vi "tvac_gui_chamber.vi"() -> ()   [LabVIEW 2016]
uses:
  <vilib>/httpClient/LabVIEWHTTPClient.lvlib
  <vilib>/httpClient/ClientHandle.ctl
  msg7171_linux.llb/send single message.vi
  <vilib>/httpClient/POSTBuffer.vi
panel:
  out "headers":string
  in  "ThermalProfile":bool
  in  "Read Zones":bool
  out "value":cluster{"ZoneSetPoint":dbl[], "ZoneTemp":dbl[]}
  out "output cluster":T1
  out "Cluster":T2
  in  "Custom Graph Selector":i32
  in  "exit":bool
  in  "AlarmColor":u32(colorbox)
  in  "Alarm String":string
  in  "Plot Color":u32(colorbox)=16860
  in  "Temperature":dbl format="%#_13g"
  in  "TC Label":string
  in  "Graph ON/OFF":u32(colorbox)=4250624
  in  "index (col)":i32
  in  "index (row)":i32
  out "working array":bool[](array[boolean])
  in  "Local Debug":bool
  in  "Tab Control":enum32{"TCs", "Graphs", "Thermal Profile"}(tab)
  in  "Log/Linear Y-Axis":u16(ring) items=["Linear", "Log"]
  in  "Total Time":dbl
  in  "Set Time TC Graph":bool
  in  "Graphing Selection":u16(ring) items=["User Selection", "Graph All Thermocouples", "Clear Graph"]
  in  "Time Scale":u16(ring) items=["Minutes", "Hours", "Seconds"]
  out "Waveform Chart":waveform(dbl)[](graph)
  out "Thermocouples":T3(array[cluster])
  in  "Log/Linear Y-Axis 6":u16(ring) items=["Linear", "Log"]
  in  "Log/Linear Y-Axis 5":u16(ring) items=["Linear", "Log"]
  in  "Log/Linear Y-Axis 3":u16(ring) items=["Linear", "Log"]
  in  "Log/Linear Y-Axis 2":u16(ring) items=["Linear", "Log"]
  in  "Total Time 6":dbl
  in  "Set Time TC Graph 6":bool
  in  "Time Scale 6":u16(ring) items=["Minutes", "Hours", "Seconds"]
  in  "Total Time 5":dbl
  in  "Set Time TC Graph 5":bool
  in  "Time Scale 5":u16(ring) items=["Minutes", "Hours", "Seconds"]
  in  "Total Time 4":dbl
  in  "Set Time TC Graph 4":bool
  in  "Time Scale 4":u16(ring) items=["Minutes", "Hours", "Seconds"]
  in  "Total Time 3":dbl
  in  "Set Time TC Graph 3":bool
  in  "Time Scale 3":u16(ring) items=["Minutes", "Hours", "Seconds"]
  in  "Total Time 2":dbl
  in  "Set Time TC Graph 2":bool
  in  "Time Scale 2":u16(ring) items=["Minutes", "Hours", "Seconds"]
  in  "Log/Linear Y-Axis 1":u16(ring) items=["Linear", "Log"]
  in  "Total Time 1":dbl
  in  "Set Time TC Graph 1":bool
  in  "Time Scale 1":u16(ring) items=["Minutes", "Hours", "Seconds"]
  in  "Custom Chart 2 Selection":i32[](listbox)=[0]
  in  "Custom Chart 1 Selection":i32[](listbox)=[0]
  out "Custom Chart 1":waveform(dbl)[](graph)
  in  "Custom Chart 3 Selection":i32[](listbox)=[0]
  in  "Custom Chart 4 Selection":i32[](listbox)=[0]
  in  "Custom Chart 5 Selection":i32[](listbox)=[0]
  in  "Custom Chart 6 Selection":i32[](listbox)=[0]
  out "Custom Chart 2":waveform(dbl)[](graph)
  out "Custom Chart 3":waveform(dbl)[](graph)
  out "Custom Chart 4":waveform(dbl)[](graph)
  out "Custom Chart 5":waveform(dbl)[](graph)
  out "Custom Chart 6":waveform(dbl)[](graph)
  in  "Log/Linear Y-Axis 4":u16(ring) items=["Linear", "Log"]
  in  "Run Profile 2":bool
  in  "Run Profile":bool
  in  "Resume Profile":bool
  in  "Stop Profile":bool
  in  "Pause Profile":bool
  in  "Hold Profile":bool
  in  "Set Z 1":bool
  in  "Z3 Thermal Profile":i32(listbox)
  in  "Z2 Thermal Profile":i32(listbox)
  in  "Z1 Thermal Profile":i32(listbox)
  in  "Zone 3 Temp":u16(ring) items=["Average", "Minimum", "Maximum"]
  in  "Zone 2 Temp":u16(ring) items=["Average", "Minimum", "Maximum"]
  in  "Zone 1 Temp":u16(ring) items=["Average", "Minimum", "Maximum"]
  in  "Zone 1 TC":i32[](listbox)=[0]
  in  "Zone 2 TC":i32[](listbox)=[0]
  in  "Zone 3 TC":i32[](listbox)=[0]
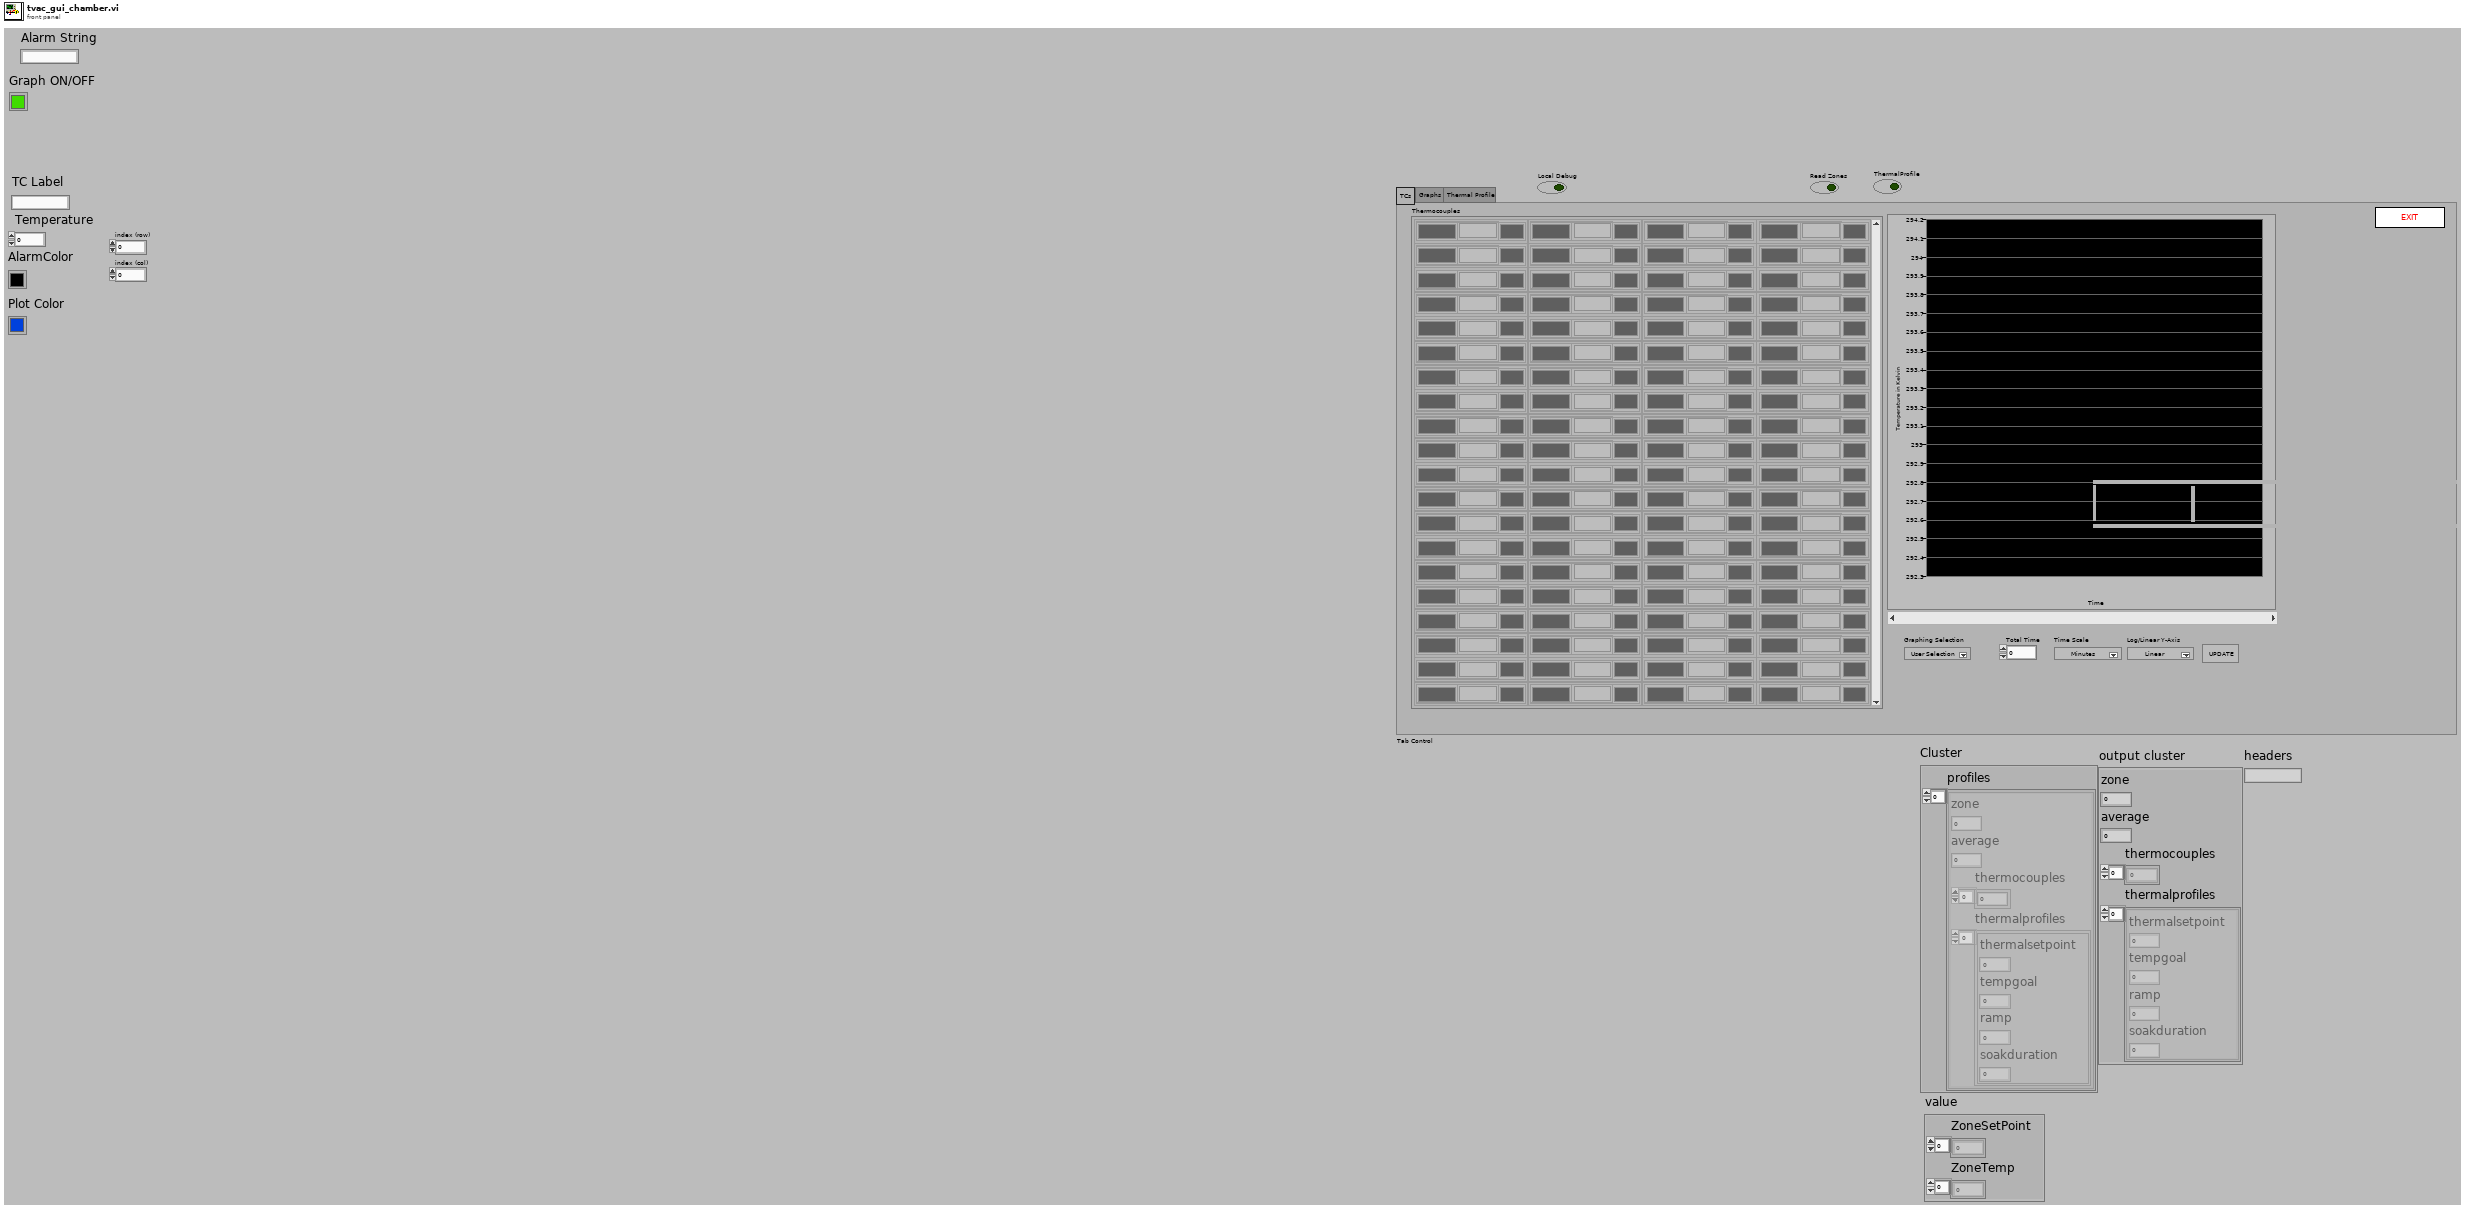
[diagram p1: front panel]
types:
  T1 = cluster{"zone":i32, "average":i32, "thermocouples":dbl[], "thermalprofiles":cluster{"thermalsetpoint":i32, "tempgoal":i32, "ramp":i32, "soakduration":i32}[]}
  T2 = cluster{"profiles":cluster{"zone":i32, "average":i32, "thermocouples":dbl[], "thermalprofiles":cluster{"thermalsetpoint":i32, "tempgoal":i32, "ramp":i32, "soakduration":i32}[]}[]}
  T3 = cluster{"TC Label":string, "Alarm Status":string, "Alarm Color":u32, "Temperature":string, "PlotColor":u32, "Graph On/Off":u32}[][]
  T4 = cluster{"thermocouple":i32, "time":dbl, "temp":dbl, "working":bool, "alarm":i32}[]
  T5 = cluster{"Cp Stage 1 Temp":dbl[], "Cp Stage 2 Temp":dbl[], "Compressor Temp":dbl[]}
  T6 = typedef "LabVIEWHTTPClient.lvlib/ClientHandle.ctl" = refnum<k1>
  T7 = cluster{"go":bool, "Http session":T6, "URL prefex":string, "index (row)":i32, "index (col)":i32, "Graph ON/OFF":u32, "TC Label":string, "Temperature":dbl, "AlarmColor":u32, "Plot Color":u32, "Alarm String":string, "Thermocouples":cluster{"TC Label":string, "Alarm Status":string, "Alarm Color":u32, "Temperature":string, "PlotColor":u32, "Graph On/Off":u32}[][], "working array":bool[], "i":i32, "NumberTCs":i32, "Waveform Chart":waveform(dbl)[], "Custom Chart 1":waveform(dbl)[], "Pressure":dbl[], "numSensors":i32, "Database":dbl[], "PumpTemps":cluster{"Cp Stage 1 Temp":dbl[], "Cp Stage 2 Temp":dbl[], "Compressor Temp":dbl[]}, "Zones":dbl[], "Time":i32, "TCs":cluster{"thermocouple":i32, "time":dbl, "temp":dbl, "working":bool, "alarm":i32}[]}
  T8 = cluster{"TC Label":string, "Alarm Status":string, "Alarm Color":u32, "Temperature":string, "PlotColor":u32, "Graph On/Off":u32}
  T9 = cluster{"CryoPressure":dbl, "ChamberPressure":dbl, "RoughingPressure":dbl}
  T10 = cluster{"time":string, "TCs":cluster{"thermocouple":i32, "time":dbl, "temp":dbl, "working":bool, "alarm":i32}[]}
  T11 = cluster{"DutyCycle":i32, "Stage1Temp":i32, "CryoPumpReadyState":cluster{"MotorOn":bool, "Ready":bool}, "PurgeValveState":bool, "RegenError":string, "RegenStep":string, "RoughingValveState":bool, "RoughingInterlock":cluster{"RoughingPermission":bool, "RoughingNeeded":bool, "Cryopumprunning":bool}, "Stage2Temp":i32, "Status":cluster{"PumpOn":bool, "RoughOpen":bool, "PurgeOpen":bool, "ThermocoupleGaugeOn":bool, "PowerFailureOccurred":bool}, "TcPressure":i32}
  T12 = typedef "LVPositionTypeDef.ctl" = cluster{"Left":i32, "Top":i32}
  T13 = typedef "LVPoint32TypeDef.ctl" = cluster{"Horizontal":i32, "Vertical":i32}
  T14 = typedef "LVRangeTypeDef.ctl" = cluster{"Minimum":dbl, "Maximum":dbl, "Increment":dbl, "Minor Increment":dbl, "Start":dbl}
  T15 = cluster{"zone":i32, "average":i32, "thermocouples":dbl[], "thermalprofiles":cluster{"thermalsetpoint":i32, "tempgoal":i32, "ramp":i32, "soakduration":i32}[]}[]
  T16 = cluster{"profiles[0]":cluster{"zone":i32, "average":i32, "thermocouples":dbl[], "thermalprofiles":cluster{"thermalsetpoint":i32, "tempgoal":i32, "ramp":i32, "soakduration":i32}[]}, "profiles[1]":cluster{"zone":i32, "average":i32, "thermocouples":dbl[], "thermalprofiles":cluster{"thermalsetpoint":i32, "tempgoal":i32, "ramp":i32, "soakduration":i32}[]}, "profiles[2]":cluster{"zone":i32, "average":i32, "thermocouples":dbl[], "thermalprofiles":cluster{"thermalsetpoint":i32, "tempgoal":i32, "ramp":i32, "soakduration":i32}[]}, "profiles[3]":cluster{"zone":i32, "average":i32, "thermocouples":dbl[], "thermalprofiles":cluster{"thermalsetpoint":i32, "tempgoal":i32, "ramp":i32, "soakduration":i32}[]}, "profiles[4]":cluster{"zone":i32, "average":i32, "thermocouples":dbl[], "thermalprofiles":cluster{"thermalsetpoint":i32, "tempgoal":i32, "ramp":i32, "soakduration":i32}[]}, "profiles[5]":cluster{"zone":i32, "average":i32, "thermocouples":dbl[], "thermalprofiles":cluster{"thermalsetpoint":i32, "tempgoal":i32, "ramp":i32, "soakduration":i32}[]}, "profiles[6]":cluster{"zone":i32, "average":i32, "thermocouples":dbl[], "thermalprofiles":cluster{"thermalsetpoint":i32, "tempgoal":i32, "ramp":i32, "soakduration":i32}[]}, "profiles[7]":cluster{"zone":i32, "average":i32, "thermocouples":dbl[], "thermalprofiles":cluster{"thermalsetpoint":i32, "tempgoal":i32, "ramp":i32, "soakduration":i32}[]}, "profiles[8]":cluster{"zone":i32, "average":i32, "thermocouples":dbl[], "thermalprofiles":cluster{"thermalsetpoint":i32, "tempgoal":i32, "ramp":i32, "soakduration":i32}[]}}
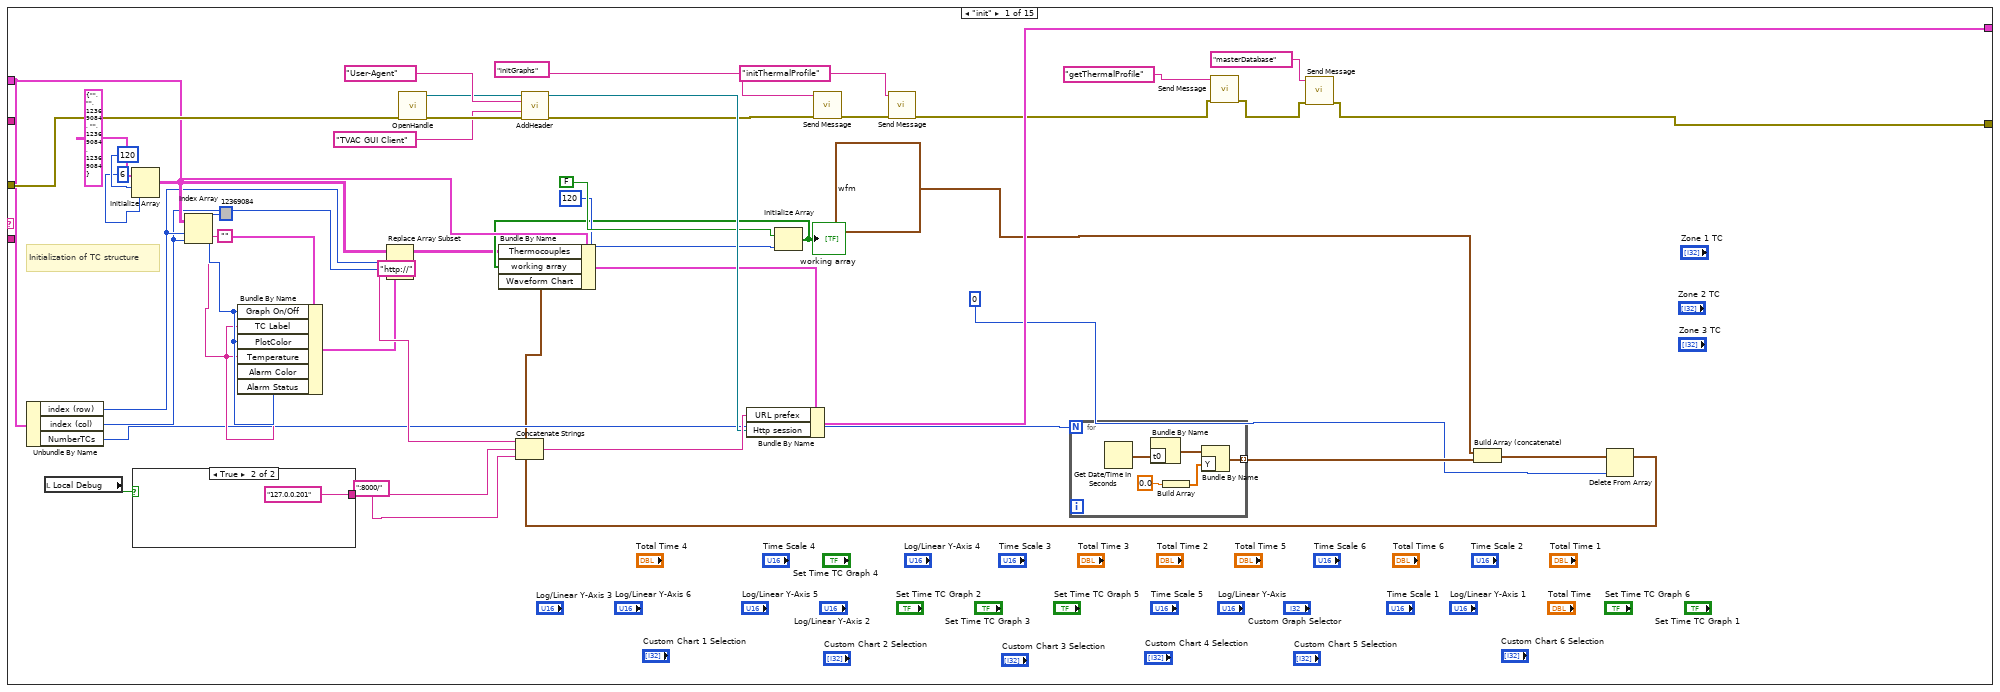
[diagram p2: hidden frame]
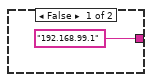
[diagram p3: hidden frame]
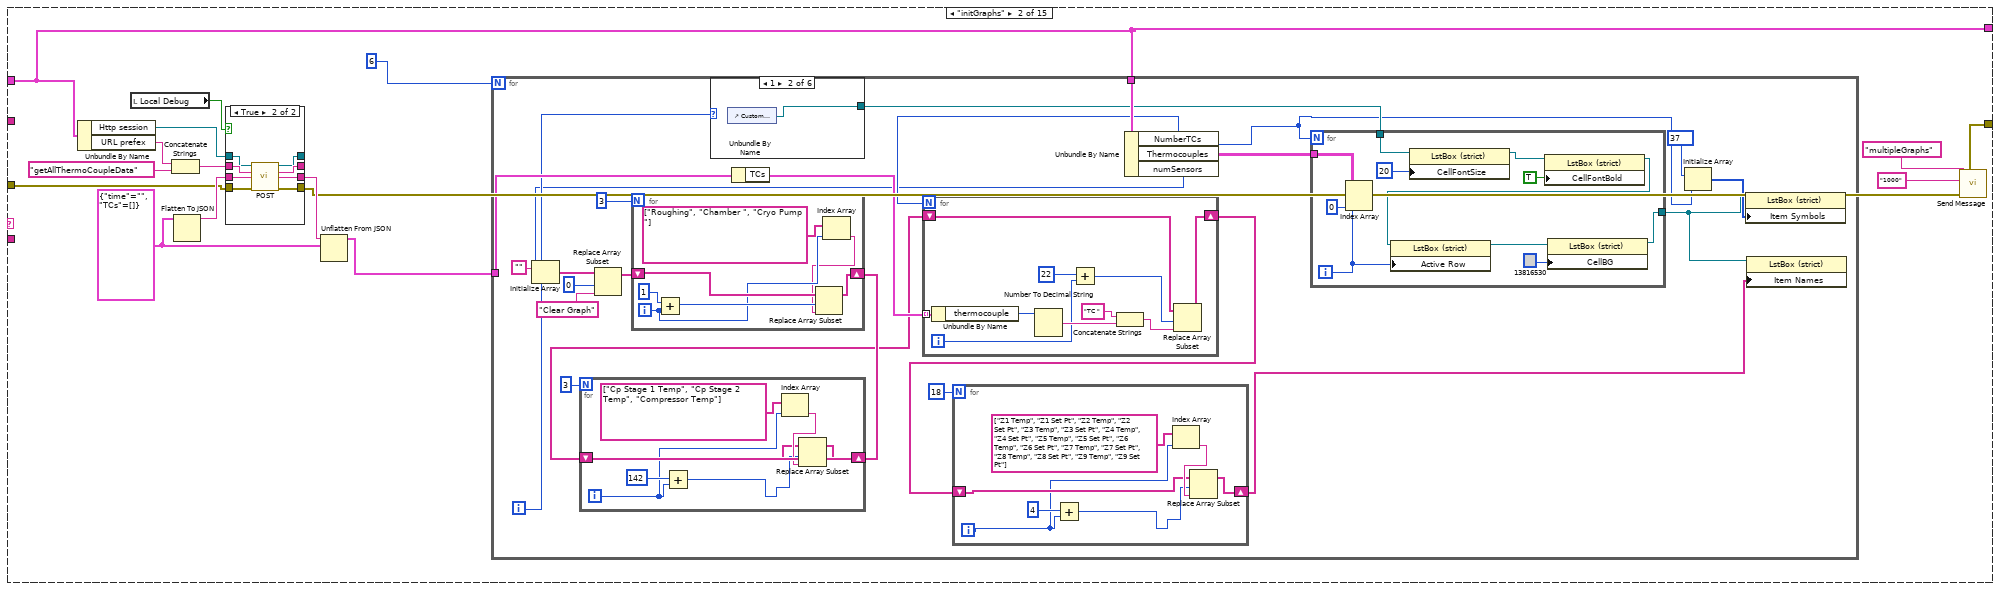
[diagram p4: hidden frame]
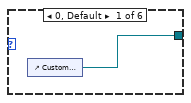
[diagram p5: hidden frame]
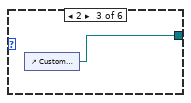
[diagram p6: hidden frame]
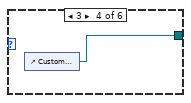
[diagram p7: hidden frame]
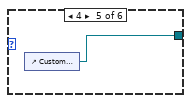
[diagram p8: hidden frame]
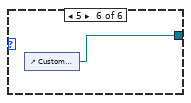
[diagram p9: hidden frame]
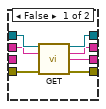
[diagram p10: hidden frame]
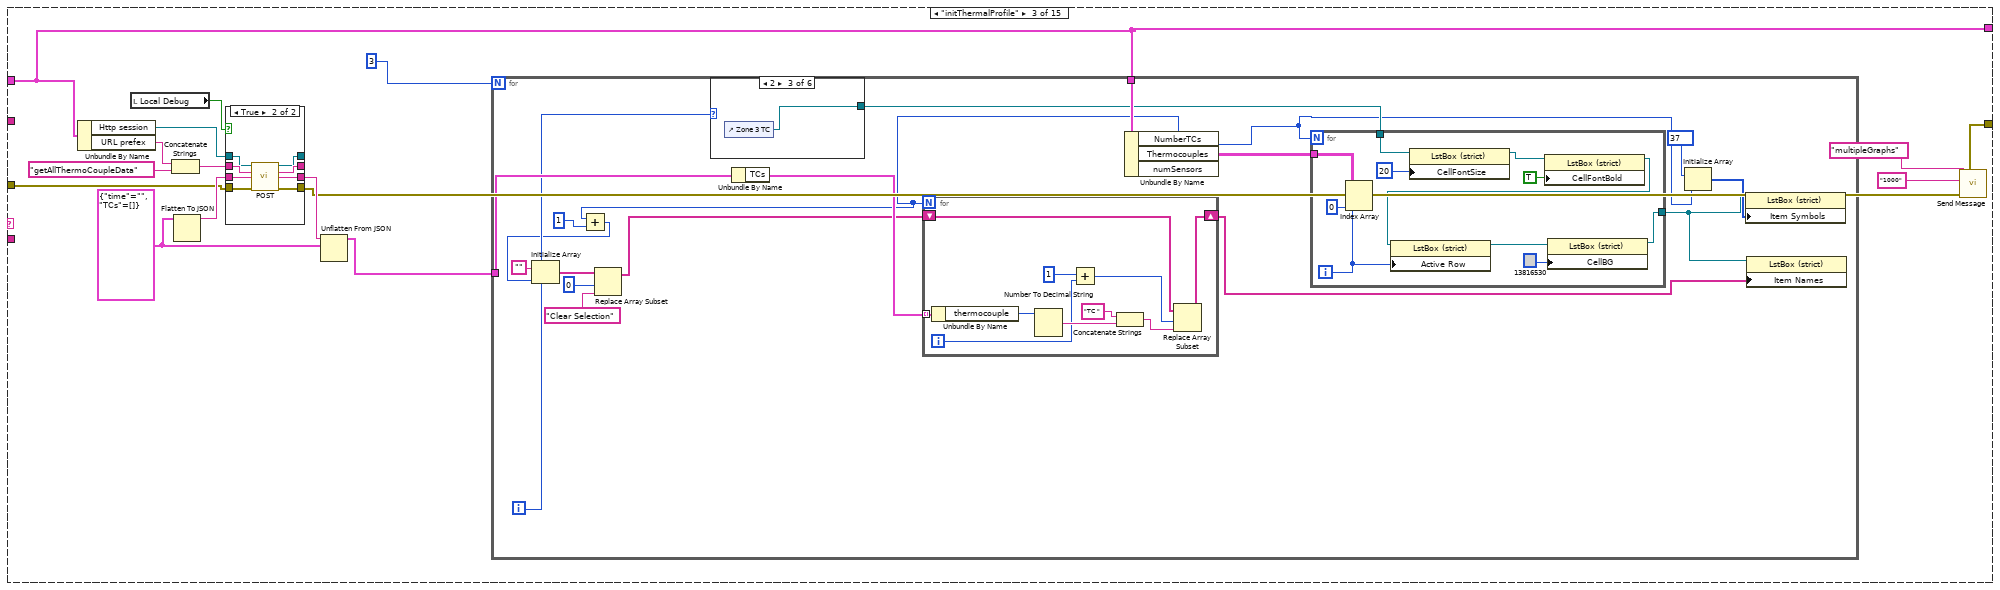
[diagram p11: hidden frame]
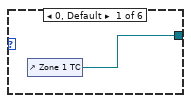
[diagram p12: hidden frame]
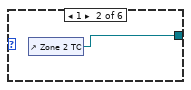
[diagram p13: hidden frame]
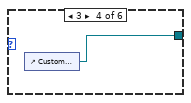
[diagram p14: hidden frame]
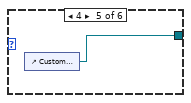
[diagram p15: hidden frame]
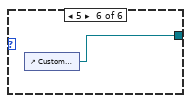
[diagram p16: hidden frame]
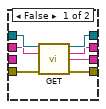
[diagram p17: hidden frame]
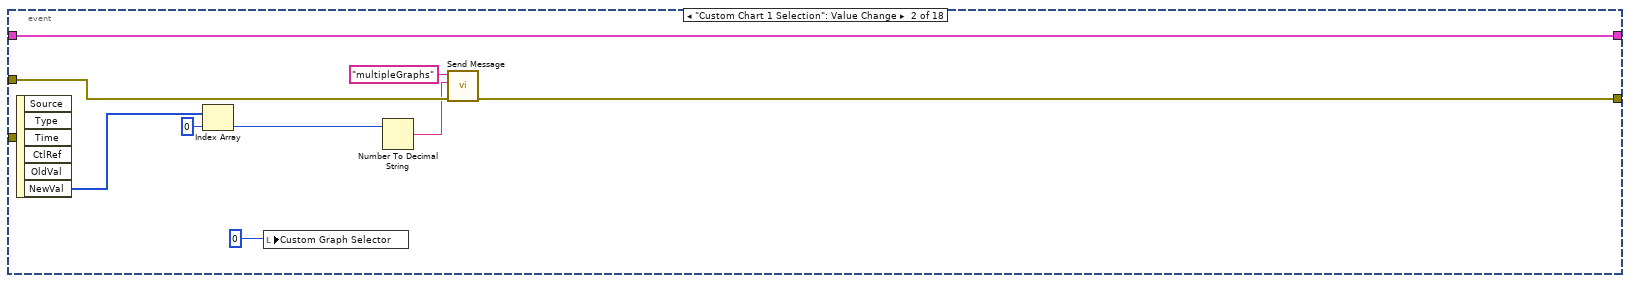
[diagram p18: hidden frame]
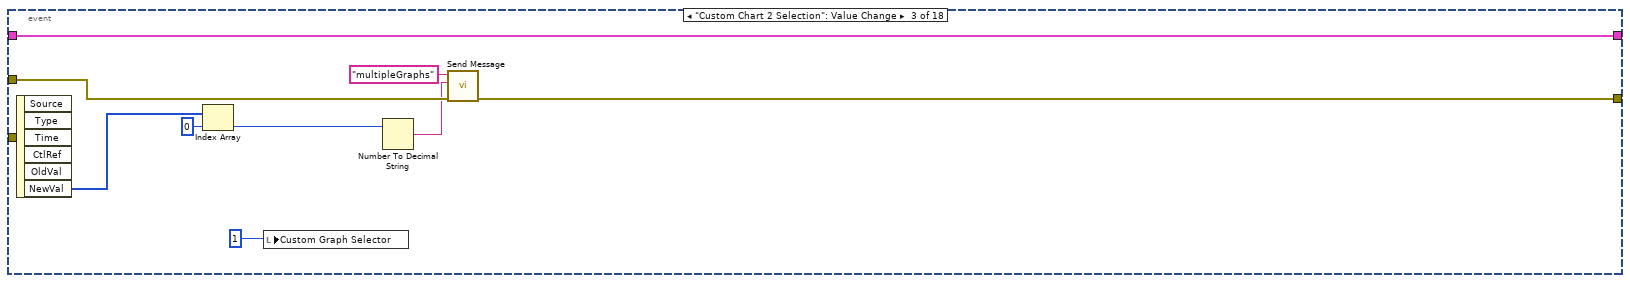
[diagram p19: hidden frame]
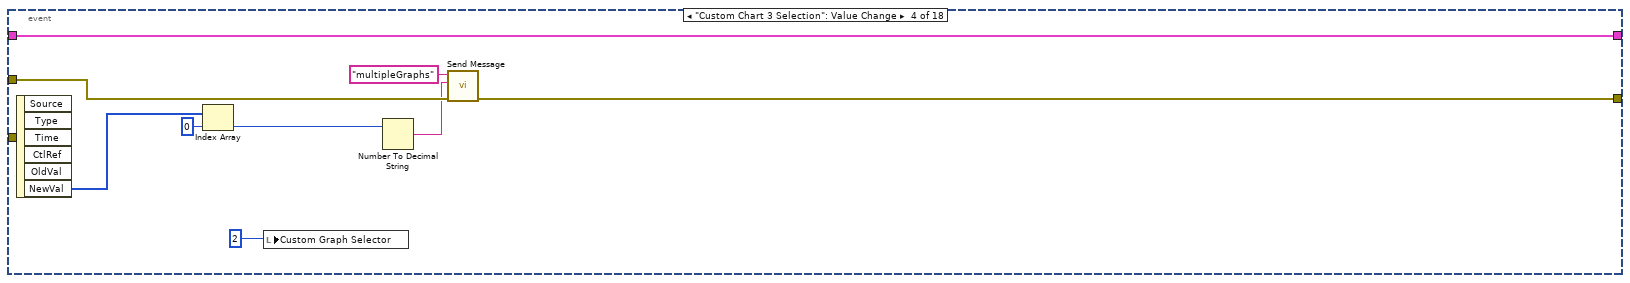
[diagram p20: hidden frame]
diagram:
  w5 = T5 {"Cp Stage 1 Temp"=[0.0], "Cp Stage 2 Temp"=[0.0], "Compressor Temp"=[0.0]}  # PumpTemps
  w8 = dbl[] [0.0, 0.0, 0.0]  # Pressure
  w28 = ""  # URL prefex
  w29 = T6 refnum  # Http session
  w30 = TRUE  # go
  n1 = call "Register Module.vi"() -> ("error out"=w26:errorcluster)  [unwired: 10 in, 1 out]
  n2 = call-poly "Send Message.vi"("error in (no error)"=w26, "event"="init") -> ("error out"=w25:errorcluster)  [unwired: 9 in]
  n3 = local read "Waveform Chart"() -> (w12:waveform(dbl)[])
  n4 = local read "Thermocouples"() -> (w10:T3)
  n5 = local read "Custom Chart 1"() -> (w9:waveform(dbl)[])
  n6 = Bundle("go"=w30, "Http session"=w29, "URL prefex"=w28, "index (row)"="index (row)", "index (col)"="index (col)", "Graph ON/OFF"="Graph ON/OFF", "TC Label"="TC Label", "Temperature"="Temperature", "AlarmColor"="AlarmColor", "Plot Color"="Plot Color", "Alarm String"="Alarm String", "Thermocouples"=w10, "working array"=bool[] [TRUE, TRUE, TRUE, TRUE, TRUE, TRUE, TRUE, TRUE, TRUE, TRUE, TRUE, TRUE, TRUE, TRUE, TRUE, TRUE, TRUE, TRUE, TRUE, TRUE, TRUE, TRUE, TRUE, TRUE, TRUE, TRUE, TRUE, TRUE, TRUE, TRUE, TRUE, TRUE, TRUE, TRUE, TRUE, TRUE, TRUE, TRUE, TRUE, TRUE, TRUE, TRUE, TRUE, TRUE, TRUE, TRUE, TRUE, TRUE, TRUE, TRUE, TRUE, TRUE, TRUE, TRUE, TRUE, TRUE, TRUE, TRUE, TRUE, TRUE, TRUE, TRUE, TRUE, TRUE, TRUE, TRUE, TRUE, TRUE, TRUE, TRUE, TRUE, TRUE, TRUE, TRUE, TRUE, TRUE, TRUE, TRUE, TRUE, TRUE, TRUE, TRUE, TRUE, TRUE, TRUE, TRUE, TRUE, TRUE, TRUE, TRUE, TRUE, TRUE, TRUE, TRUE, TRUE, TRUE, TRUE, TRUE, TRUE, TRUE, TRUE, TRUE, TRUE, TRUE, TRUE, TRUE, TRUE, TRUE, TRUE, TRUE, TRUE, TRUE, TRUE, TRUE, TRUE, TRUE, TRUE, TRUE, TRUE, TRUE], "i"=0, "NumberTCs"=120, "Waveform Chart"=w12, "Custom Chart 1"=w9, "Pressure"=w8, "numSensors"=145, "Database"=dbl[] [0.0, 1000.5841582194602, 1000.5841582194602, 1000.5841582194602, 0.6389895835935778, 0.7578061575842531, 1.153531014677555, 1.4572061556343079, 1.0192558642672256, 0.9245021790184325, 0.34311035179988925, 1.1970333160202968, 1.066989851322369, 0.5926593131154867, 0.7219240511326698, 1.0529790116491695, 1.4485694746891444, 0.9139060201605569, 0.7997359753068659, 0.6568795179977746, 0.8470104541419833, 1.0272585161866683, 0.6577301535824354, 0.645139941938139, 1.5235316442408067, 0.5128651184775285, 1.6421980587090137, 1.3961508335147417, 1.1242639015795428, 1.5954313466624428, 1.1919135255187876, 1.2615004458206727, 1.1320092264321664, 1.922759836270222, 1.1315561200367314, 1.4924621723754858, 0.6988771274186227, 1.069709701591943, 0.9920698240997152, 0.5395549253287656, 0.42891479657680576, 1.2794224940227927, 0.2687949632437338, 0.16127136772755854, 1.0174597006256374, 1.2079238230365172, 0.9745554383837218, 1.5348516925460962, 0.9488878852839246, 1.6634477658652282, 1.1924291951744272, 1.2231949298067308, 1.2223766746774598, 1.30664154589907, 1.2872878364107239, 0.5274250065177812, 0.7905999067114673, 1.2748974665085449, 1.216972941585413, 0.959115576325391, 0.5743502840762814, 0.8219540421676025, 0.613053899308251, 1.3785560870413707, 1.034117232127813, 1.1237698659753859, 1.4495548642149667, 0.6967905980938514, 0.6224497255665377, 1.6551326273040576, 1.2103048396824558, 0.6078721016951973, 1.3790669246280296, 0.5454332940871525, 1.5318777012492035, 1.2496539590411258, 0.9145395304446965, 1.3855381787793546, 1.0857600342029163, 1.3185833631438346, 0.9769688683142593, 1.026663691242448, 0.6744610422623843, 1.1965175398567691, 0.4847084945450119, 0.6435799980029115, 0.8079659363810663, 0.9130053929540112, 0.5271098423006861, 0.8088111736464799, 1.1455315536576556, 1.139809531926708, 1.5840192673434794, 1.0296748968089129, 1.7370669751200136, 1.3715484550405317, 0.3362063953932494, 1.0385868418202253, 1.4947740276021626, 1.0393600693910505, 0.8870410800672984, 1.2470388696569872, 0.9846724980375481, 0.9952471377109308, 1.0807485178906029, 1.1016630607035562, 1.3301039036808464, 0.8856852816151205, 0.4719509873120426, 0.5191430277856135, 0.12135113366044793, 0.4230478635224125, 1.1140562049976255, 1.5484968368781251, 1.1999891199114734, 1.8721302183420216, 1.071489235222563, 0.6260864330445979, 1.0305668002030492, 1.0223711899566386, 0.7842533472819472, 1.7301290335750898, 1.318694748426881, 0.6978662965493679], "PumpTemps"=w5, "Zones"=dbl[] [24.54828257301887, 25.0, 20.035959453954195, 26.0, 28.926820041278148, 27.0, 21.321976066931608, 28.0, 29.197600688359813, 29.0, 29.117373424110085, 30.0, 21.092914485312942, 31.0, 27.791581465649088, 32.0, 24.70861457288988, 33.0], "Time"=0, "TCs"=T4 []) -> (w16:T7)  [unwired: 1 in]
  n7 = call "getData.vi"("Local Debug"=TRUE) -> ()  [unwired: 11 in]
  n8 = while {
    shift-left: w16 -> [w35]
    shift-right: [w32] -> _
    shift-right: [w33] -> w11
    shift-left: w25 -> [w40]
    stop <- w31 continue-if-true
    n9 = call "Get Message.vi"("error in (no error)"=w40) -> ("error out"=w38:errorcluster, "event buffer"=w39:string, "event"=w37:string, "source"=w36:string)  [unwired: 7 in]
    n10 = case shown="\"\", \"Idle\"" w37 {
      selector: w37 -> [_ _ _ _ _ _ _ _ _ _ _ _ _ _ w1344]
      tunnel: [w76 w97 w199 w281 w968 w975 w1051 w1078 w1082 w1122 w1176 w1196 w1327 w1342 w1346] -> w32
      tunnel: w35 -> [w57 w97 w199 w282 w969 w980 w1055 w1073 w1082 w1118 w1177 w1196 w1327 w1338 w1346]
      tunnel: w39 -> [_ _ _ _ w960 _ w1054 _ _ _ _ w1197 _ _ _]
      tunnel: w38 -> [w79 w96 w198 w270 w961 w970 w1052 w1058 w1080 w1123 w1182 _ _ w1341 w1345]
      tunnel: [w42 w92 w194 w280 w961 w970 w1052 w1058 w1080 w1123 w1182 _ _ w1340 w1343] -> w34
      tunnel: w36 -> [_ _ _ _ _ _ _ _ _ _ _ _ _ _ _]
      frame "init" {
        w62 = ""
        w63 = u32 12369084 ("PlotColor")
        # "Initialization of TC structure"
        n11 = Unbundle By Name(w57) -> ("index (row)"=w65:i32, "index (col)"=w64:i32, "NumberTCs"=w54:i32)
        n12 = local read "Local Debug"() -> (w70:bool)
        n13 = Initialize Array(T8 {"TC Label"="", "Alarm Status"="", "Alarm Color"=12369084, "Temperature"="", "PlotColor"=12369084, "Graph On/Off"=12369084}, 120 ("dimension size"), 6 ("dimension size")) -> (w66:T3)
        n14 = case shown="True" w70 {
          tunnel: ["192.168.99.1" ("Address") "127.0.0.201" ("Address")] -> w71
          frame False {
          }
          frame True {
          }
        }
        n15 = Index Array(array=w66, index (row)=w65, index (col)=w64) -> (element=w61:T8)
        n16 = Bundle By Name(cluster=w61, "Graph On/Off"=w63, "TC Label"=w62, "PlotColor"=w63, "Temperature"=w62, "Alarm Color"=w63, "Alarm Status"=w62) -> (w60:T8)
        n17 = Replace Array Subset(array=w66, new element=w60, index (row)=w65, index (col)=w64) -> (w48:T3)
        n18 = call <vilib>:"OpenHandle.vi"("error in (no error)"=w79) -> ("client handle out"=w80:T6, "error out"=w83:errorcluster)  [unwired: 13 in]
        n19 = Concatenate Strings("http://" ("url"), w71, ":8000/" ("url")) -> (w75:string)
        n20 = call <vilib>:"AddHeader.vi"("client handle"=w80, "header"="User-Agent", "value"="TVAC GUI Client", "error in (no error)"=w83) -> ("client handle out"=w74:T6, "error out"=w73:errorcluster)  [unwired: 10 in]
        n21 = Initialize Array(FALSE ("Boolean"), 120 ("dimension size")) -> (w55:bool[])
        "working array" <- w55
        n22 = call-poly "Send Message.vi"("error in (no error)"=w73, "event"="initGraphs") -> ("error out"=w47:errorcluster)  [unwired: 9 in]
        n23 = call-poly "Send Message.vi"("error in (no error)"=w47, "event"="initThermalProfile") -> ("error out"=w45:errorcluster)  [unwired: 9 in]
        n24 = for {
          N: w54 -> [_]
          tunnel: [w84] -> w52 mode=indexing
          n25 = Get Date/Time In Seconds() -> (seconds since 1Jan1904=w88:timestamp)
          n26 = Bundle By Name("t0"=w88) -> (w85:waveform(dbl))  [unwired: 1 in]
          n27 = Build Array(0.0) -> (w87:dbl[])
          n28 = Bundle By Name(cluster=w85, "Y"=w87) -> (w84:waveform(dbl))
        }
        n29 = call-poly "Send Message.vi"("error in (no error)"=w45, "event"="getThermalProfile") -> ("error out"=w43:errorcluster)  [unwired: 9 in]
        n30 = call-poly "Send Message.vi"("error in (no error)"=w43, "event"="masterDatabase") -> ("error out"=w42:errorcluster)  [unwired: 9 in]
        n31 = Build Array (concatenate)(waveform(dbl) {"t0"=timestamp(0 s since 1904-01-01), "dt"=1.0, "Y"=[0.0]} ("element"), w52) -> (w53:waveform(dbl)[])
        n32 = Delete From Array(array=w53, index=0) -> (array with subset deleted=w51:waveform(dbl)[])  [unwired: 1 in, 1 out]
        n33 = Bundle By Name(cluster=w57, "Thermocouples"=w48, "working array"=w55, "Waveform Chart"=w51) -> (w56:T7)
        n34 = Bundle By Name(cluster=w56, "URL prefex"=w75, "Http session"=w74) -> (w76:T7)
      }
      frame "initGraphs" {
        w100 = T10 {"time"="", "TCs"=[]} ("Cluster")
        n35 = Unbundle By Name(w97) -> ("Http session"=w106:T6, "URL prefex"=w104:string)
        n36 = local read "Local Debug"() -> (w98:bool)
        n37 = Concatenate Strings(w104, "getAllThermoCoupleData" ("url")) -> (w105:string)
        n38 = Flatten To JSON(anything=w100) -> (JSON string=w99:string)  [unwired: 2 in, 1 out]
        n39 = case shown="True" w98 {
          tunnel: w96 -> [w184 w185]
          tunnel: [w183 w186] -> w93
          tunnel: [w182 w187] -> _
          tunnel: w106 -> [w181 w190]
          tunnel: w105 -> [w180 w191]
          tunnel: [w179 w188] -> w102
          tunnel: [w178 w189] -> _
          tunnel: w99 -> [_ w192]
          frame False {
            n40 = call <vilib>:"GET.vi"("client handle"=w181, "url"=w180, "error in (no error)"=w184) -> ("client handle out"=w182:T6, "headers"=w178:string, "body"=w179:string, "error out"=w183:errorcluster)  [unwired: 9 in]
          }
          frame True {
            n41 = call-poly <vilib>:"POST.vi"("client handle"=w190, "url"=w191, "buffer"=w192, "error in (no error)"=w185) -> ("client handle out"=w187:T6, "headers"=w189:string, "body"=w188:string, "error out"=w186:errorcluster)  [unwired: 8 in]
          }
        }
        n42 = Unflatten From JSON(JSON string=w102, type and defaults=w100) -> (value=w101:T10)  [unwired: 5 in, 1 out]
        n43 = for {
          N: 6 ("Numeric") -> [_]
          tunnel: w101 -> [w128]
          tunnel: w97 -> [w127]
          i -> [w110]
          n44 = case shown="1" w110 {
            tunnel: [w130 w131 w132 w133 w134 w135] -> w111
            frame 0, Default {
              n45 = control-ref of="Custom Chart 1 Selection"() -> (w130:refnum<vi>)
            }
            frame 1 {
              n46 = control-ref of="Custom Chart 2 Selection"() -> (w131:refnum<vi>)
            }
            frame 2 {
              n47 = control-ref of="Custom Chart 3 Selection"() -> (w132:refnum<vi>)
            }
            frame 3 {
              n48 = control-ref of="Custom Chart 4 Selection"() -> (w133:refnum<vi>)
            }
            frame 4 {
              n49 = control-ref of="Custom Chart 5 Selection"() -> (w134:refnum<vi>)
            }
            frame 5 {
              n50 = control-ref of="Custom Chart 6 Selection"() -> (w135:refnum<vi>)
            }
          }
          n51 = Unbundle By Name(w128) -> ("TCs"=w124:T4)
          n52 = Unbundle By Name(w127) -> ("NumberTCs"=w122:i32, "Thermocouples"=w129:T3, "numSensors"=w108:i32)
          n53 = Initialize Array("", w108) -> (w120:string[])
          n54 = Replace Array Subset(array=w120, new element="Clear Graph" ("new element/subarray"), index=0) -> (w117:string[])
          n55 = for {
            N: 3 -> [_]
            shift-right: [w155] -> w115
            shift-left: w117 -> [w156]
            i -> [w151]
            n56 = Add(x=1 ("index"), y=w151) -> (x+y=w153:i32)
            n57 = Index Array(array=string[] ["Roughing", "Chamber ", "Cryo Pump "], index=w151) -> (element=w150:string)
            n58 = Replace Array Subset(array=w156, new element=w150, index=w153) -> (w155:string[])
          }
          n59 = for {
            N: 3 -> [_]
            shift-right: [w146] -> w114
            shift-left: w115 -> [w147]
            i -> [w143]
            n60 = Add(x=142 ("index"), y=w143) -> (x+y=w144:i32)
            n61 = Index Array(array=string[] ["Cp Stage 1 Temp", "Cp Stage 2 Temp", "Compressor Temp"], index=w143) -> (element=w148:string)
            n62 = Replace Array Subset(array=w147, new element=w148, index=w144) -> (w146:string[])
          }
          n63 = for {
            N: w122 -> [_]
            tunnel: w124 -> [w163] mode=indexing
            shift-right: [w157] -> w107
            shift-left: w114 -> [w159]
            i -> [w161]
            n64 = Unbundle By Name(w163) -> ("thermocouple"=w164:i32)
            n65 = Number To Decimal String(number=w164) -> (decimal integer string=w166:string)  [unwired: 1 in]
            n66 = Add(x=22 ("index"), y=w161) -> (x+y=w160:i32)
            n67 = Concatenate Strings("TC " ("string"), w166) -> (w158:string)
            n68 = Replace Array Subset(array=w159, new element=w158, index=w160) -> (w157:string[])
          }
          n69 = for {
            N: 18 -> [_]
            shift-right: [w136] -> w113
            shift-left: w107 -> [w138]
            i -> [w137]
            n70 = Add(x=4 ("index"), y=w137) -> (x+y=w139:i32)
            n71 = Index Array(array=string[] ["Z1 Temp", "Z1 Set Pt", "Z2 Temp", "Z2 Set Pt", "Z3 Temp", "Z3 Set Pt", "Z4 Temp", "Z4 Set Pt", "Z5 Temp", "Z5 Set Pt", "Z6 Temp", "Z6 Set Pt", "Z7 Temp", "Z7 Set Pt", "Z8 Temp", "Z8 Set Pt", "Z9 Temp", "Z9 Set Pt"], index=w137) -> (element=w141:string)
            n72 = Replace Array Subset(array=w138, new element=w141, index=w139) -> (w136:string[])
          }
          n73 = for {
            N: w108 -> [_]
            tunnel: w129 -> [w177]
            tunnel: w111 -> [w171]
            tunnel: [w167] -> w109
            i -> [w174]
            n74 = Index Array(array=w177, index (row)=w174, index (col)=0 ("disabled index (col)")) -> ()  [unwired: 1 out]
            n75 = property on="Property Node" class="LstBox (strict)"(reference=w171, "CellFontSize"=u32 20 ("Active Row:Cell Font:Size")) -> (reference out=w170:refnum<vi>)  [unwired: 1 in, 1 out]
            n76 = property on="Property Node" class="LstBox (strict)"(reference=w170, "CellFontBold"=TRUE ("Active Row:Cell Font:Bold")) -> (reference out=w169:refnum<vi>)  [unwired: 1 in, 1 out]
            n77 = property on="Property Node" class="LstBox (strict)"(reference=w169, "Active Row"=w174) -> (reference out=w168:refnum<vi>)  [unwired: 1 in, 1 out]
            n78 = property on="Property Node" class="LstBox (strict)"(reference=w168, "CellBG"=u32 13816530 ("Active Row:Cell Background Color")) -> (reference out=w167:refnum<vi>)  [unwired: 1 in, 1 out]
          }
          n79 = Initialize Array(37, w108) -> (w125:i32[])
          n80 = property on="Property Node" class="LstBox (strict)"(reference=w109, "Item Symbols"=w125) -> ()  [unwired: 1 in, 2 out]
          n81 = property on="Property Node" class="LstBox (strict)"(reference=w109, "Item Names"=w113) -> ()  [unwired: 1 in, 2 out]
        }
        n82 = call-poly "Send Message.vi"("error in (no error)"=w93, "event buffer"="1000", "event"="multipleGraphs") -> ("error out"=w92:errorcluster)  [unwired: 8 in]
      }
      frame "initThermalProfile" {
        w202 = T10 {"time"="", "TCs"=[]} ("Cluster")
        n83 = Unbundle By Name(w199) -> ("Http session"=w208:T6, "URL prefex"=w206:string)
        n84 = local read "Local Debug"() -> (w200:bool)
        n85 = Concatenate Strings(w206, "getAllThermoCoupleData" ("url")) -> (w207:string)
        n86 = Flatten To JSON(anything=w202) -> (JSON string=w201:string)  [unwired: 2 in, 1 out]
        n87 = case shown="True" w200 {
          tunnel: w198 -> [w261 w262]
          tunnel: [w260 w263] -> w195
          tunnel: [w259 w264] -> _
          tunnel: w208 -> [w258 w267]
          tunnel: w207 -> [w257 w268]
          tunnel: [w256 w265] -> w204
          tunnel: [w255 w266] -> _
          tunnel: w201 -> [_ w269]
          frame False {
            n88 = call <vilib>:"GET.vi"("client handle"=w258, "url"=w257, "error in (no error)"=w261) -> ("client handle out"=w259:T6, "headers"=w255:string, "body"=w256:string, "error out"=w260:errorcluster)  [unwired: 9 in]
          }
          frame True {
            n89 = call-poly <vilib>:"POST.vi"("client handle"=w267, "url"=w268, "buffer"=w269, "error in (no error)"=w262) -> ("client handle out"=w264:T6, "headers"=w266:string, "body"=w265:string, "error out"=w263:errorcluster)  [unwired: 8 in]
          }
        }
        n90 = Unflatten From JSON(JSON string=w204, type and defaults=w202) -> (value=w203:T10)  [unwired: 5 in, 1 out]
        n91 = for {
          N: 3 ("Numeric") -> [_]
          tunnel: w203 -> [w226]
          tunnel: w199 -> [w225]
          i -> [w216]
          n92 = case shown="2" w216 {
            tunnel: [w228 w229 w230 w231 w232 w233] -> w217
            frame 0, Default {
              n93 = control-ref of="Zone 1 TC"() -> (w228:refnum<vi>)
            }
            frame 1 {
              n94 = control-ref of="Zone 2 TC"() -> (w229:refnum<vi>)
            }
            frame 2 {
              n95 = control-ref of="Zone 3 TC"() -> (w230:refnum<vi>)
            }
            frame 3 {
              n96 = control-ref of="Custom Chart 4 Selection"() -> (w231:refnum<vi>)
            }
            frame 4 {
              n97 = control-ref of="Custom Chart 5 Selection"() -> (w232:refnum<vi>)
            }
            frame 5 {
              n98 = control-ref of="Custom Chart 6 Selection"() -> (w233:refnum<vi>)
            }
          }
          n99 = Unbundle By Name(w226) -> ("TCs"=w222:T4)
          n100 = Unbundle By Name(w225) -> ("NumberTCs"=w211:i32, "Thermocouples"=w227:T3, "numSensors"=w214:i32)
          n101 = Add(x=w211, y=1 ("index")) -> (x+y=w209:i32)
          n102 = Initialize Array("", w209) -> (w220:string[])
          n103 = Replace Array Subset(array=w220, new element="Clear Selection" ("new element/subarray"), index=0) -> (w213:string[])
          n104 = for {
            N: w211 -> [_]
            tunnel: w222 -> [w240] mode=indexing
            shift-right: [w234] -> w212
            shift-left: w213 -> [w236]
            i -> [w238]
            n105 = Unbundle By Name(w240) -> ("thermocouple"=w241:i32)
            n106 = Number To Decimal String(number=w241) -> (decimal integer string=w243:string)  [unwired: 1 in]
            n107 = Add(x=1 ("index"), y=w238) -> (x+y=w237:i32)
            n108 = Concatenate Strings("TC " ("string"), w243) -> (w235:string)
            n109 = Replace Array Subset(array=w236, new element=w235, index=w237) -> (w234:string[])
          }
          n110 = for {
            N: w214 -> [_]
            tunnel: w227 -> [w254]
            tunnel: w217 -> [w248]
            tunnel: [w244] -> w215
            i -> [w251]
            n111 = Index Array(array=w254, index (row)=w251, index (col)=0 ("disabled index (col)")) -> ()  [unwired: 1 out]
            n112 = property on="Property Node" class="LstBox (strict)"(reference=w248, "CellFontSize"=u32 20 ("Active Row:Cell Font:Size")) -> (reference out=w247:refnum<vi>)  [unwired: 1 in, 1 out]
            n113 = property on="Property Node" class="LstBox (strict)"(reference=w247, "CellFontBold"=TRUE ("Active Row:Cell Font:Bold")) -> (reference out=w246:refnum<vi>)  [unwired: 1 in, 1 out]
            n114 = property on="Property Node" class="LstBox (strict)"(reference=w246, "Active Row"=w251) -> (reference out=w245:refnum<vi>)  [unwired: 1 in, 1 out]
            n115 = property on="Property Node" class="LstBox (strict)"(reference=w245, "CellBG"=u32 13816530 ("Active Row:Cell Background Color")) -> (reference out=w244:refnum<vi>)  [unwired: 1 in, 1 out]
          }
          n116 = Initialize Array(37, w214) -> (w223:i32[])
          n117 = property on="Property Node" class="LstBox (strict)"(reference=w215, "Item Symbols"=w223) -> ()  [unwired: 1 in, 2 out]
          n118 = property on="Property Node" class="LstBox (strict)"(reference=w215, "Item Names"=w212) -> ()  [unwired: 1 in, 2 out]
        }
        n119 = call-poly "Send Message.vi"("error in (no error)"=w195, "event buffer"="1000", "event"="multipleGraphs") -> ("error out"=w194:errorcluster)  [unwired: 8 in]
      }
      frame "", "Idle" {
        n120 = control-ref of="Thermocouples"() -> (w279:refnum<vi>)
        n121 = property on="Property Node" class="Arr (strict)"(reference=w279) -> ("Position"=w278:T12)  [unwired: 1 in, 2 out]
        n122 = Unbundle By Name(w278) -> ("Left"=w277:i32, "Top"=w275:i32)
        n123 = Add(x=4, y=w277) -> (x+y=w273:i32)
        n124 = Add(x=w275, y=23 ("x")) -> (x+y=w272:i32)
        n125 = event shown="[0] Timeout" {
          selector: _ -> [_ _ _ _ _ _ _ _ _ _ _ _ _ _ _ _ _ _]
          dyn-events: _ -> [_ _ _ _ _ _ _ _ _ _ _ _ _ _ _ _ _ _]
          timeout: 200 ("milliseconds to wait") -> [_ _ _ _ _ _ _ _ _ _ _ _ _ _ _ _ _ _]
          tunnel: w270 -> [_ w311 w320 w329 w338 w347 w356 w361 w376 w469 w533 w594 w655 w716 w777 w838 w899 w958]
          tunnel: [w305 w310 w319 w328 w337 w346 w355 w360 w376 w469 w533 w594 w655 w716 w777 w838 w899 w956] -> w280
          tunnel: [w298 w312 w321 w330 w339 w348 w357 w365 w377 w463 w534 w595 w656 w717 w778 w839 w900 w959] -> w281
          tunnel: w282 -> [w299 w312 w321 w330 w339 w348 w357 w365 w378 w465 w534 w595 w656 w717 w778 w839 w900 w959]
          tunnel: w273 -> [_ _ _ _ _ _ _ _ w375 _ _ _ _ _ _ _ _ _]
          tunnel: w272 -> [_ _ _ _ _ _ _ _ w372 _ _ _ _ _ _ _ _ _]
          tunnel: w270 -> [w294 _ _ _ _ _ _ _ _ _ _ _ _ _ _ _ _ _]
          event Timeout {
            n126 = event-data() -> ("Time"=w297:u32)  [unwired: 1 in, 1 out]
            n127 = Unbundle By Name(w299) -> ("Time"=w302:i32)
            n128 = Subtract(x=w297, y=w302) -> (x-y=w301:u32)
            n129 = Greater?(x=w301, y=u32 1000 ("millisecond multiple")) -> ()  [unwired: 1 out]
            n130 = Bundle By Name(cluster=w299, "Time"=w297) -> (w298:T7)
            n131 = call-poly "Send Message.vi"("Destination Module"="getData.vi", "error in (no error)"=w294, "event"="getTC") -> ("error out"=w287:errorcluster)  [unwired: 8 in]
            n132 = call-poly "Send Message.vi"("Destination Module"="getData.vi", "error in (no error)"=w287, "event"="getPressure") -> ("error out"=w283:errorcluster)  [unwired: 8 in]
            n133 = call-poly "Send Message.vi"("Destination Module"="getData.vi", "error in (no error)"=w283, "event"="getMCCData") -> ("error out"=w296:errorcluster)  [unwired: 8 in]
            n134 = call-poly "Send Message.vi"("error in (no error)"=w296, "event"="masterDatabase") -> ("error out"=w293:errorcluster)  [unwired: 9 in]
            n135 = call-poly "Send Message.vi"("error in (no error)"=w293, "event"="graphTC") -> ("error out"=w292:errorcluster)  [unwired: 9 in]
            n136 = call-poly "Send Message.vi"("error in (no error)"=w292, "event buffer"="1000", "event"="multipleGraphs") -> ("error out"=w305:errorcluster)  [unwired: 8 in]
          }
          event "Custom Chart 1 Selection": Value Change {
            n137 = event-data() -> ("NewVal"=w313:i32[])  [unwired: 1 in, 5 out]
            n138 = Index Array(array=w313, index=0) -> (element=w307:i32)
            n139 = local write "Custom Graph Selector"(0) -> ()
            n140 = Number To Decimal String(number=w307) -> (decimal integer string=w308:string)  [unwired: 1 in]
            n141 = call-poly "Send Message.vi"("error in (no error)"=w311, "event buffer"=w308, "event"="multipleGraphs") -> ("error out"=w310:errorcluster)  [unwired: 8 in]
          }
          event "Custom Chart 2 Selection": Value Change {
            n142 = event-data() -> ("NewVal"=w322:i32[])  [unwired: 1 in, 5 out]
            n143 = Index Array(array=w322, index=0) -> (element=w316:i32)
            n144 = local write "Custom Graph Selector"(1) -> ()
            n145 = Number To Decimal String(number=w316) -> (decimal integer string=w317:string)  [unwired: 1 in]
            n146 = call-poly "Send Message.vi"("error in (no error)"=w320, "event buffer"=w317, "event"="multipleGraphs") -> ("error out"=w319:errorcluster)  [unwired: 8 in]
          }
          event "Custom Chart 3 Selection": Value Change {
            n147 = event-data() -> ("NewVal"=w331:i32[])  [unwired: 1 in, 5 out]
            n148 = Index Array(array=w331, index=0) -> (element=w325:i32)
            n149 = local write "Custom Graph Selector"(2) -> ()
            n150 = Number To Decimal String(number=w325) -> (decimal integer string=w326:string)  [unwired: 1 in]
            n151 = call-poly "Send Message.vi"("error in (no error)"=w329, "event buffer"=w326, "event"="multipleGraphs") -> ("error out"=w328:errorcluster)  [unwired: 8 in]
          }
          event "Custom Chart 4 Selection": Value Change {
            n152 = event-data() -> ("NewVal"=w340:i32[])  [unwired: 1 in, 5 out]
            n153 = Index Array(array=w340, index=0) -> (element=w334:i32)
            n154 = local write "Custom Graph Selector"(3) -> ()
            n155 = Number To Decimal String(number=w334) -> (decimal integer string=w335:string)  [unwired: 1 in]
            n156 = call-poly "Send Message.vi"("error in (no error)"=w338, "event buffer"=w335, "event"="multipleGraphs") -> ("error out"=w337:errorcluster)  [unwired: 8 in]
          }
          event "Custom Chart 5 Selection": Value Change {
            n157 = event-data() -> ("NewVal"=w349:i32[])  [unwired: 1 in, 5 out]
            n158 = Index Array(array=w349, index=0) -> (element=w343:i32)
            n159 = local write "Custom Graph Selector"(4) -> ()
            n160 = Number To Decimal String(number=w343) -> (decimal integer string=w344:string)  [unwired: 1 in]
            n161 = call-poly "Send Message.vi"("error in (no error)"=w347, "event buffer"=w344, "event"="multipleGraphs") -> ("error out"=w346:errorcluster)  [unwired: 8 in]
          }
          event "Custom Chart 6 Selection": Value Change {
            n162 = event-data() -> ("NewVal"=w358:i32[])  [unwired: 1 in, 5 out]
            n163 = Index Array(array=w358, index=0) -> (element=w352:i32)
            n164 = local write "Custom Graph Selector"(5) -> ()
            n165 = Number To Decimal String(number=w352) -> (decimal integer string=w353:string)  [unwired: 1 in]
            n166 = call-poly "Send Message.vi"("error in (no error)"=w356, "event buffer"=w353, "event"="multipleGraphs") -> ("error out"=w355:errorcluster)  [unwired: 8 in]
          }
          event "Tab Control": Value Change {
            n167 = event-data() -> ("NewVal"=w364:enum32{"TCs", "Graphs", "Thermal Profile"})  [unwired: 1 in, 5 out]
            n168 = Equal?(x=w364, y=enum16{"Graphs"}."Graphs") -> (x = y?=w362:bool)
            n169 = case shown="True" w362 {
              tunnel: w361 -> [w366 w368]
              tunnel: [w366 w367] -> w360
              frame False {
              }
              frame True {
                n170 = call-poly "Send Message.vi"("error in (no error)"=w368, "event"="getGraphs") -> ("error out"=w367:errorcluster)  [unwired: 9 in]
              }
            }
          }
          event "Thermocouples": Mouse Down {
            n171 = event-data() -> ("CtlRef"=w380:refnum<vi>, "Coords"=w385:T13)  [unwired: 1 in, 3 out]
            n172 = Unbundle By Name(w385) -> ("Horizontal"=w383:i32, "Vertical"=w382:i32)
            n173 = Add(x=783 ("y"), y=w375) -> (x+y=w370:i32)
            n174 = Less?(x=w383, y=w370) -> (x < y?=w384:bool)
            n175 = Add(x=w372, y=854) -> (x+y=w371:i32)
            n176 = Less?(x=w382, y=w371) -> (x < y?=w381:bool)
            n177 = And(x=w384, y=w381) -> (x .and. y?=w379:bool)
            n178 = case shown="True" w379 {
              tunnel: w380 -> [_ w427]
              tunnel: w378 -> [_ w399]
              tunnel: w378 -> [w386 w397]
              tunnel: [w386 w389] -> w377
              tunnel: w375 -> [_ w388]
              tunnel: w372 -> [_ w387]
              frame False {
              }
              frame True {
                w421 = u16 0 items=["User Selection", "Graph All Thermocouples", "Clear Graph"] ("Graphing Selection")
                n179 = property class="Arr (strict)"(reference=w427) -> ("Array Element.Position"=w419:T12)  [unwired: 1 in, 2 out]
                n180 = local write "Graphing Selection"(w421) -> ()
                n181 = Unbundle By Name(w419) -> ("Left"=w417:i32, "Top"=w420:i32)
                n182 = property on="Thermocouples" class="Arr (strict)"() -> ("Index Values"=w411:u32[])  [unwired: 2 in, 2 out]
                n183 = Subtract(x=w388, y=w417) -> (x-y=w416:i32)
                n184 = Subtract(x=w387, y=w420) -> (x-y=w408:i32)
                n185 = Absolute Value(x=w408) -> (abs(x)=w418:i32)
                n186 = Index Array(array=w411, index=0) -> (element=w407:u32)
                n187 = To Byte Integer(number=w407) -> (8bit integer=w406:i8)
                n188 = Absolute Value(x=w416) -> (abs(x)=w415:i32)
                n189 = local read "Thermocouples"() -> (w390:T3)
                n190 = Quotient & Remainder(x=w418, y=42) -> (floor(x/y)=w405:i32)  [unwired: 1 out]
                n191 = Add(x=w406, y=w405) -> (x+y=w392:i32)
                n192 = Quotient & Remainder(x=w415, y=197 ("Numeric 2")) -> (floor(x/y)=w391:i32)  [unwired: 1 out]
                n193 = Index Array(array=w390, index (row)=w392, index (col)=w391) -> (element=w393:T8)
                n194 = Multiply(x=4, y=w392) -> (x*y=w412:i32)
                n195 = Unbundle By Name(w399) -> ("working array"=w398:bool[])  [unwired: 1 out]
                n196 = Unbundle By Name(w393) -> ("Alarm Color"=w425:u32, "Graph On/Off"=w424:u32, "TC Label"=w423:string, "PlotColor"=w404:u32, "Alarm Status"=w422:string, "Temperature"=w395:string)
                n197 = Add(x=w412, y=w391) -> (x+y=w401:i32)
                n198 = control-ref of="Waveform Chart"() -> (w426:refnum<vi>)
                n199 = Index Array(array=w398, index=w401) -> (element=w400:bool)
                n200 = Decimal String To Number(string=w395) -> ()  [unwired: 2 in, 2 out]
                n201 = Equal?(x=w424, y=u32 12369084) -> (x = y?=w402:bool)
                n202 = case shown="True" w400 {
                  selector: w400 -> [_ w433]
                  tunnel: w426 -> [_ w439]
                  tunnel: w425 -> [_ w438]
                  tunnel: w423 -> [_ w437]
                  tunnel: w422 -> [_ w436]
                  tunnel: w401 -> [_ w429]
                  tunnel: w404 -> [_ w435]
                  tunnel: w402 -> [_ w434]
                  tunnel: w395 -> [_ w432]
                  tunnel: [w428 w431] -> w394
                  tunnel: w393 -> [w428 w430]
                  frame False {
                  }
                  frame True {
                    n203 = case shown="True" w434 {
                      tunnel: w439 -> [w449 w460]
                      tunnel: w438 -> [w443 w455]
                      tunnel: w437 -> [w444 w454]
                      tunnel: w436 -> [w445 w456]
                      tunnel: w435 -> [_ w458]
                      tunnel: w433 -> [_ _]
                      tunnel: w432 -> [w446 w457]
                      tunnel: [w441 w453] -> w431
                      tunnel: w430 -> [w442 w452]
                      tunnel: w429 -> [w440 w451]
                      frame False {
                        w447 = u32 12369084
                        n204 = property on="Property Node" class="WFChart (strict)"(reference=w449, "Active Plot"=w440) -> (reference out=w450:refnum<vi>)  [unwired: 1 in, 1 out]
                        n205 = Bundle By Name(cluster=w442, "Graph On/Off"=w447, "TC Label"=w444, "PlotColor"=w447, "Temperature"=w446, "Alarm Color"=w443, "Alarm Status"=w445) -> (w441:T8)
                        n206 = property class="WFChart (strict)"(reference=w450, "Plot.Visible?"=FALSE ("Plot.Visible")) -> ()  [unwired: 1 in, 2 out]
                      }
                      frame True {
                        n207 = property class="WFChart (strict)"(reference=w460, "Active Plot"=w451) -> (reference out=w461:refnum<vi>)  [unwired: 1 in, 1 out]
                        n208 = Bundle By Name(cluster=w452, "Graph On/Off"=u32 6618880, "TC Label"=w454, "PlotColor"=w458, "Temperature"=w457, "Alarm Color"=w455, "Alarm Status"=w456) -> (w453:T8)
                        n209 = property class="WFChart (strict)"(reference=w461, "Plot.Visible?"=TRUE ("Plot.Visible")) -> ()  [unwired: 1 in, 2 out]
                      }
                    }
                  }
                }
                n210 = Replace Array Subset(array=w390, new element=w394, index (row)=w392, index (col)=w391) -> (w396:T3)
                n211 = Bundle By Name(cluster=w397, "Thermocouples"=w396) -> (w389:T7)
              }
            }
          }
          event "Graphing Selection": Value Change {
            n212 = event-data() -> ("NewVal"=w470:u16)  [unwired: 1 in, 5 out]
            n213 = Unbundle By Name(w465) -> ("Thermocouples"=w464:T3, "working array"=w467:bool[])
            n214 = control-ref of="Waveform Chart"() -> (w471:refnum<vi>)
            n215 = case shown="1" w470 {
              tunnel: w464 -> [w472 w477 w508]
              tunnel: w471 -> [_ w476 w507]
              tunnel: 120 ("disabled index (col)") -> [_ w475 w506]
              tunnel: w465 -> [_ _ _]
              tunnel: w467 -> [_ w474 _]
              tunnel: [w472 w473 w505] -> w466
              frame 0, Default {
              }
              frame 1 {
                n216 = for {
                  N: w475 -> [_]
                  tunnel: w476 -> [w483]
                  shift-right: [w478] -> w473
                  shift-left: w477 -> [w482]
                  tunnel: w474 -> [w479]
                  i -> [w481]
                  n217 = Index Array(array=w479, index=w481) -> (element=w480:bool)
                  n218 = case shown="True" w480 {
                    tunnel: w483 -> [_ w504]
                    tunnel: w482 -> [w484 w485]
                    tunnel: [w484 w486] -> w478
                    tunnel: w481 -> [_ w503]
                    frame False {
                    }
                    frame True {
                      n219 = Quotient & Remainder(x=w503, y=4) -> (x-y*floor(x/y)=w489:i32, floor(x/y)=w488:i32)
                      n220 = Multiply(x=4, y=w488) -> (x*y=w499:i32)
                      n221 = Add(x=w499, y=w489) -> (x+y=w498:i32)
                      n222 = property class="WFChart (strict)"(reference=w504, "Active Plot"=w498) -> (reference out=w501:refnum<vi>)  [unwired: 1 in, 1 out]
                      n223 = Index Array(array=w485, index (row)=w488, index (col)=w489) -> (element=w487:T8)
                      n224 = Unbundle By Name(w487) -> ("TC Label"=w490:string, "Alarm Status"=w496:string, "Temperature"=w495:string, "PlotColor"=w492:u32, "Alarm Color"=w491:u32)
                      n225 = property class="WFChart (strict)"(reference=w501, "Plot.Visible?"=TRUE ("Plot.Visible")) -> ()  [unwired: 1 in, 2 out]
                      n226 = Bundle By Name(cluster=w487, "TC Label"=w490, "Alarm Status"=w496, "Alarm Color"=w491, "Temperature"=w495, "PlotColor"=w492, "Graph On/Off"=u32 6618880) -> (w494:T8)
                      n227 = Replace Array Subset(array=w485, new element=w494, index (row)=w488, index (col)=w489) -> (w486:T3)
                    }
                  }
                }
              }
              frame 2 {
                n228 = for {
                  N: w506 -> [_]
                  tunnel: w507 -> [w526]
                  shift-right: [w509] -> w505
                  shift-left: w508 -> [w513]
                  i -> [w527]
                  w519 = u32 12369084
                  n229 = local read "working array"() -> (w528:bool[])
                  n230 = Quotient & Remainder(x=w527, y=4 ("Numeric")) -> (x-y*floor(x/y)=w511:i32, floor(x/y)=w510:i32)
                  n231 = Index Array(array=w513, index (row)=w510, index (col)=w511) -> (element=w518:T8)
                  n232 = Multiply(x=4, y=w510) -> (x*y=w522:i32)
                  n233 = Add(x=w522, y=w511) -> (x+y=w521:i32)
                  n234 = Index Array(array=w528, index=w527) -> ()  [unwired: 1 out]
                  n235 = property class="WFChart (strict)"(reference=w526, "Active Plot"=w521) -> (reference out=w524:refnum<vi>)  [unwired: 1 in, 1 out]
                  n236 = Unbundle By Name(w518) -> ("TC Label"=w517:string, "Alarm Status"=w516:string, "Temperature"=w515:string, "PlotColor"=w514:u32)
                  n237 = property class="WFChart (strict)"(reference=w524, "Plot.Visible?"=FALSE ("Plot.Visible")) -> ()  [unwired: 1 in, 2 out]
                  n238 = Bundle By Name(cluster=w518, "TC Label"=w517, "Alarm Status"=w516, "Alarm Color"=w519, "Temperature"=w515, "PlotColor"=w514, "Graph On/Off"=w519) -> (w512:T8)
                  n239 = Replace Array Subset(array=w513, new element=w512, index (row)=w510, index (col)=w511) -> (w509:T3)
                }
              }
            }
            n240 = Bundle By Name(cluster=w465, "Thermocouples"=w466) -> (w463:T7)
          }
          event "Set Time TC Graph": Mouse Down {
            n241 = event-data() -> ()  [unwired: 1 in, 8 out]
            n242 = local read "Log/Linear Y-Axis"() -> (w530:u16)
            n243 = control-ref of="Waveform Chart"() -> (w529:refnum<vi>)
            n244 = property on="Property Node" class="WFChart (strict)"(reference=w529, "YScale.Mapping Mode"=w530) -> ()  [unwired: 1 in, 2 out]
            n245 = local read "Total Time"() -> (w531:dbl)
            n246 = local read "Time Scale"() -> (w532:u16)
            n247 = case shown="2" w532 {
              tunnel: w529 -> [w537 w556 w575]
              tunnel: w531 -> [w535 w554 w573]
              frame 0, Default {
                n248 = Not Equal To 0?(x=w535) -> (x != 0?=w536:bool)
                n249 = case shown="True" w536 {
                  tunnel: w537 -> [w539 w551]
                  tunnel: w535 -> [_ w545]
                  frame False {
                    n250 = property on="Property Node" class="WFChart (strict)"(reference=w539) -> (reference out=w538:refnum<vi>, "XScale.Range"=w544:T14)  [unwired: 1 in, 1 out]
                    n251 = Bundle By Name(cluster=w544, "Minimum"=0.0, "Maximum"=3600.0, "Increment"=60.0) -> (w543:T14)
                    n252 = property on="Property Node" class="WFChart (strict)"(reference=w538, "XScale.Range"=w543) -> ()  [unwired: 1 in, 2 out]
                  }
                  frame True {
                    n253 = property on="Property Node" class="WFChart (strict)"(reference=w551) -> (reference out=w548:refnum<vi>, "XScale.Range"=w553:T14)  [unwired: 1 in, 1 out]
                    n254 = Multiply(x=w545, y=60.0) -> (x*y=w547:dbl)
                    n255 = Bundle By Name(cluster=w553, "Minimum"=0.0, "Maximum"=w547, "Increment"=1.0) -> (w552:T14)
                    n256 = property on="Property Node" class="WFChart (strict)"(reference=w548, "XScale.Range"=w552) -> ()  [unwired: 1 in, 2 out]
                  }
                }
              }
              frame 1 {
                n257 = Not Equal To 0?(x=w554) -> (x != 0?=w555:bool)
                n258 = case shown="True" w555 {
                  tunnel: w556 -> [w558 w568]
                  tunnel: w554 -> [_ w565]
                  frame False {
                    n259 = property on="Property Node" class="WFChart (strict)"(reference=w558) -> (reference out=w557:refnum<vi>, "XScale.Range"=w563:T14)  [unwired: 1 in, 1 out]
                    n260 = Bundle By Name(cluster=w563, "Minimum"=0.0, "Maximum"=43200.0, "Increment"=3600.0) -> (w559:T14)
                    n261 = property on="Property Node" class="WFChart (strict)"(reference=w557, "XScale.Range"=w559) -> ()  [unwired: 1 in, 2 out]
                  }
                  frame True {
                    n262 = Multiply(x=w565, y=3600.0) -> (x*y=w564:dbl)
                    n263 = property on="Property Node" class="WFChart (strict)"(reference=w568) -> (reference out=w567:refnum<vi>, "XScale.Range"=w572:T14)  [unwired: 1 in, 1 out]
                    n264 = Bundle By Name(cluster=w572, "Minimum"=0.0, "Maximum"=w564, "Increment"=3600.0) -> (w569:T14)
                    n265 = property on="Property Node" class="WFChart (strict)"(reference=w567, "XScale.Range"=w569) -> ()  [unwired: 1 in, 2 out]
                  }
                }
              }
              frame 2 {
                n266 = Not Equal To 0?(x=w573) -> (x != 0?=w574:bool)
                n267 = case shown="True" w574 {
                  tunnel: w575 -> [w577 w585]
                  tunnel: w573 -> [_ w583]
                  frame False {
                    n268 = property on="Property Node" class="WFChart (strict)"(reference=w577) -> (reference out=w576:refnum<vi>, "XScale.Range"=w582:T14)  [unwired: 1 in, 1 out]
                    n269 = Bundle By Name(cluster=w582, "Minimum"=0.0, "Maximum"=60.0, "Increment"=1.0) -> (w578:T14)
                    n270 = property on="Property Node" class="WFChart (strict)"(reference=w576, "XScale.Range"=w578) -> ()  [unwired: 1 in, 2 out]
                  }
                  frame True {
                    n271 = property on="Property Node" class="WFChart (strict)"(reference=w585) -> (reference out=w584:refnum<vi>, "XScale.Range"=w589:T14)  [unwired: 1 in, 1 out]
                    n272 = Bundle By Name(cluster=w589, "Minimum"=0.0, "Maximum"=w583, "Increment"=1.0) -> (w586:T14)
                    n273 = property on="Property Node" class="WFChart (strict)"(reference=w584, "XScale.Range"=w586) -> ()  [unwired: 1 in, 2 out]
                  }
                }
              }
            }
          }
          event "Set Time TC Graph 1": Mouse Down {
            n274 = event-data() -> ()  [unwired: 1 in, 8 out]
            n275 = local read "Log/Linear Y-Axis 1"() -> (w591:u16)
            n276 = control-ref of="Custom Chart 1"() -> (w590:refnum<vi>)
            n277 = property on="Property Node" class="WFChart (strict)"(reference=w590, "YScale.Mapping Mode"=w591) -> ()  [unwired: 1 in, 2 out]
            n278 = local read "Total Time 1"() -> (w592:dbl)
            n279 = local read "Time Scale 1"() -> (w593:u16)
            n280 = case shown="2" w593 {
              tunnel: w590 -> [w598 w617 w636]
              tunnel: w592 -> [w596 w615 w634]
              frame 0, Default {
                n281 = Not Equal To 0?(x=w596) -> (x != 0?=w597:bool)
                n282 = case shown="True" w597 {
                  tunnel: w598 -> [w600 w612]
                  tunnel: w596 -> [_ w606]
                  frame False {
                    n283 = property on="Property Node" class="WFChart (strict)"(reference=w600) -> (reference out=w599:refnum<vi>, "XScale.Range"=w605:T14)  [unwired: 1 in, 1 out]
                    n284 = Bundle By Name(cluster=w605, "Minimum"=0.0, "Maximum"=3600.0, "Increment"=60.0) -> (w604:T14)
                    n285 = property on="Property Node" class="WFChart (strict)"(reference=w599, "XScale.Range"=w604) -> ()  [unwired: 1 in, 2 out]
                  }
                  frame True {
                    n286 = property on="Property Node" class="WFChart (strict)"(reference=w612) -> (reference out=w609:refnum<vi>, "XScale.Range"=w614:T14)  [unwired: 1 in, 1 out]
                    n287 = Multiply(x=w606, y=60.0) -> (x*y=w608:dbl)
                    n288 = Bundle By Name(cluster=w614, "Minimum"=0.0, "Maximum"=w608, "Increment"=1.0) -> (w613:T14)
                    n289 = property on="Property Node" class="WFChart (strict)"(reference=w609, "XScale.Range"=w613) -> ()  [unwired: 1 in, 2 out]
                  }
                }
              }
              frame 1 {
                n290 = Not Equal To 0?(x=w615) -> (x != 0?=w616:bool)
                n291 = case shown="True" w616 {
                  tunnel: w617 -> [w619 w629]
                  tunnel: w615 -> [_ w626]
                  frame False {
                    n292 = property on="Property Node" class="WFChart (strict)"(reference=w619) -> (reference out=w618:refnum<vi>, "XScale.Range"=w624:T14)  [unwired: 1 in, 1 out]
                    n293 = Bundle By Name(cluster=w624, "Minimum"=0.0, "Maximum"=43200.0, "Increment"=3600.0) -> (w620:T14)
                    n294 = property on="Property Node" class="WFChart (strict)"(reference=w618, "XScale.Range"=w620) -> ()  [unwired: 1 in, 2 out]
                  }
                  frame True {
                    n295 = Multiply(x=w626, y=3600.0) -> (x*y=w625:dbl)
                    n296 = property on="Property Node" class="WFChart (strict)"(reference=w629) -> (reference out=w628:refnum<vi>, "XScale.Range"=w633:T14)  [unwired: 1 in, 1 out]
                    n297 = Bundle By Name(cluster=w633, "Minimum"=0.0, "Maximum"=w625, "Increment"=3600.0) -> (w630:T14)
                    n298 = property on="Property Node" class="WFChart (strict)"(reference=w628, "XScale.Range"=w630) -> ()  [unwired: 1 in, 2 out]
                  }
                }
              }
              frame 2 {
                n299 = Not Equal To 0?(x=w634) -> (x != 0?=w635:bool)
                n300 = case shown="True" w635 {
                  tunnel: w636 -> [w638 w646]
                  tunnel: w634 -> [_ w644]
                  frame False {
                    n301 = property on="Property Node" class="WFChart (strict)"(reference=w638) -> (reference out=w637:refnum<vi>, "XScale.Range"=w643:T14)  [unwired: 1 in, 1 out]
                    n302 = Bundle By Name(cluster=w643, "Minimum"=0.0, "Maximum"=60.0, "Increment"=1.0) -> (w639:T14)
                    n303 = property on="Property Node" class="WFChart (strict)"(reference=w637, "XScale.Range"=w639) -> ()  [unwired: 1 in, 2 out]
                  }
                  frame True {
                    n304 = property on="Property Node" class="WFChart (strict)"(reference=w646) -> (reference out=w645:refnum<vi>, "XScale.Range"=w650:T14)  [unwired: 1 in, 1 out]
                    n305 = Bundle By Name(cluster=w650, "Minimum"=0.0, "Maximum"=w644, "Increment"=1.0) -> (w647:T14)
                    n306 = property on="Property Node" class="WFChart (strict)"(reference=w645, "XScale.Range"=w647) -> ()  [unwired: 1 in, 2 out]
                  }
                }
              }
            }
          }
          event "Set Time TC Graph 2": Mouse Down {
            n307 = event-data() -> ()  [unwired: 1 in, 8 out]
            n308 = local read "Log/Linear Y-Axis 2"() -> (w652:u16)
            n309 = control-ref of="Custom Chart 2"() -> (w651:refnum<vi>)
            n310 = property on="Property Node" class="WFChart (strict)"(reference=w651, "YScale.Mapping Mode"=w652) -> ()  [unwired: 1 in, 2 out]
            n311 = local read "Total Time 2"() -> (w653:dbl)
            n312 = local read "Time Scale 2"() -> (w654:u16)
            n313 = case shown="2" w654 {
              tunnel: w651 -> [w659 w678 w697]
              tunnel: w653 -> [w657 w676 w695]
              frame 0, Default {
                n314 = Not Equal To 0?(x=w657) -> (x != 0?=w658:bool)
                n315 = case shown="True" w658 {
                  tunnel: w659 -> [w661 w673]
                  tunnel: w657 -> [_ w667]
                  frame False {
                    n316 = property on="Property Node" class="WFChart (strict)"(reference=w661) -> (reference out=w660:refnum<vi>, "XScale.Range"=w666:T14)  [unwired: 1 in, 1 out]
                    n317 = Bundle By Name(cluster=w666, "Minimum"=0.0, "Maximum"=3600.0, "Increment"=60.0) -> (w665:T14)
                    n318 = property on="Property Node" class="WFChart (strict)"(reference=w660, "XScale.Range"=w665) -> ()  [unwired: 1 in, 2 out]
                  }
                  frame True {
                    n319 = property on="Property Node" class="WFChart (strict)"(reference=w673) -> (reference out=w670:refnum<vi>, "XScale.Range"=w675:T14)  [unwired: 1 in, 1 out]
                    n320 = Multiply(x=w667, y=60.0) -> (x*y=w669:dbl)
                    n321 = Bundle By Name(cluster=w675, "Minimum"=0.0, "Maximum"=w669, "Increment"=1.0) -> (w674:T14)
                    n322 = property on="Property Node" class="WFChart (strict)"(reference=w670, "XScale.Range"=w674) -> ()  [unwired: 1 in, 2 out]
                  }
                }
              }
              frame 1 {
                n323 = Not Equal To 0?(x=w676) -> (x != 0?=w677:bool)
                n324 = case shown="True" w677 {
                  tunnel: w678 -> [w680 w690]
                  tunnel: w676 -> [_ w687]
                  frame False {
                    n325 = property on="Property Node" class="WFChart (strict)"(reference=w680) -> (reference out=w679:refnum<vi>, "XScale.Range"=w685:T14)  [unwired: 1 in, 1 out]
                    n326 = Bundle By Name(cluster=w685, "Minimum"=0.0, "Maximum"=43200.0, "Increment"=3600.0) -> (w681:T14)
                    n327 = property on="Property Node" class="WFChart (strict)"(reference=w679, "XScale.Range"=w681) -> ()  [unwired: 1 in, 2 out]
                  }
                  frame True {
                    n328 = Multiply(x=w687, y=3600.0) -> (x*y=w686:dbl)
                    n329 = property on="Property Node" class="WFChart (strict)"(reference=w690) -> (reference out=w689:refnum<vi>, "XScale.Range"=w694:T14)  [unwired: 1 in, 1 out]
                    n330 = Bundle By Name(cluster=w694, "Minimum"=0.0, "Maximum"=w686, "Increment"=3600.0) -> (w691:T14)
                    n331 = property on="Property Node" class="WFChart (strict)"(reference=w689, "XScale.Range"=w691) -> ()  [unwired: 1 in, 2 out]
                  }
                }
              }
              frame 2 {
                n332 = Not Equal To 0?(x=w695) -> (x != 0?=w696:bool)
                n333 = case shown="True" w696 {
                  tunnel: w697 -> [w699 w707]
                  tunnel: w695 -> [_ w705]
                  frame False {
                    n334 = property on="Property Node" class="WFChart (strict)"(reference=w699) -> (reference out=w698:refnum<vi>, "XScale.Range"=w704:T14)  [unwired: 1 in, 1 out]
                    n335 = Bundle By Name(cluster=w704, "Minimum"=0.0, "Maximum"=60.0, "Increment"=1.0) -> (w700:T14)
                    n336 = property on="Property Node" class="WFChart (strict)"(reference=w698, "XScale.Range"=w700) -> ()  [unwired: 1 in, 2 out]
                  }
                  frame True {
                    n337 = property on="Property Node" class="WFChart (strict)"(reference=w707) -> (reference out=w706:refnum<vi>, "XScale.Range"=w711:T14)  [unwired: 1 in, 1 out]
                    n338 = Bundle By Name(cluster=w711, "Minimum"=0.0, "Maximum"=w705, "Increment"=1.0) -> (w708:T14)
                    n339 = property on="Property Node" class="WFChart (strict)"(reference=w706, "XScale.Range"=w708) -> ()  [unwired: 1 in, 2 out]
                  }
                }
              }
            }
          }
          event "Set Time TC Graph 3": Mouse Down {
            n340 = event-data() -> ()  [unwired: 1 in, 8 out]
            n341 = local read "Log/Linear Y-Axis 3"() -> (w713:u16)
            n342 = control-ref of="Custom Chart 3"() -> (w712:refnum<vi>)
            n343 = property on="Property Node" class="WFChart (strict)"(reference=w712, "YScale.Mapping Mode"=w713) -> ()  [unwired: 1 in, 2 out]
            n344 = local read "Total Time 3"() -> (w714:dbl)
            n345 = local read "Time Scale 3"() -> (w715:u16)
            n346 = case shown="2" w715 {
              tunnel: w712 -> [w720 w739 w758]
              tunnel: w714 -> [w718 w737 w756]
              frame 0, Default {
                n347 = Not Equal To 0?(x=w718) -> (x != 0?=w719:bool)
                n348 = case shown="True" w719 {
                  tunnel: w720 -> [w722 w734]
                  tunnel: w718 -> [_ w728]
                  frame False {
                    n349 = property on="Property Node" class="WFChart (strict)"(reference=w722) -> (reference out=w721:refnum<vi>, "XScale.Range"=w727:T14)  [unwired: 1 in, 1 out]
                    n350 = Bundle By Name(cluster=w727, "Minimum"=0.0, "Maximum"=3600.0, "Increment"=60.0) -> (w726:T14)
                    n351 = property on="Property Node" class="WFChart (strict)"(reference=w721, "XScale.Range"=w726) -> ()  [unwired: 1 in, 2 out]
                  }
                  frame True {
                    n352 = property on="Property Node" class="WFChart (strict)"(reference=w734) -> (reference out=w731:refnum<vi>, "XScale.Range"=w736:T14)  [unwired: 1 in, 1 out]
                    n353 = Multiply(x=w728, y=60.0) -> (x*y=w730:dbl)
                    n354 = Bundle By Name(cluster=w736, "Minimum"=0.0, "Maximum"=w730, "Increment"=1.0) -> (w735:T14)
                    n355 = property on="Property Node" class="WFChart (strict)"(reference=w731, "XScale.Range"=w735) -> ()  [unwired: 1 in, 2 out]
                  }
                }
              }
              frame 1 {
                n356 = Not Equal To 0?(x=w737) -> (x != 0?=w738:bool)
                n357 = case shown="True" w738 {
                  tunnel: w739 -> [w741 w751]
                  tunnel: w737 -> [_ w748]
                  frame False {
                    n358 = property on="Property Node" class="WFChart (strict)"(reference=w741) -> (reference out=w740:refnum<vi>, "XScale.Range"=w746:T14)  [unwired: 1 in, 1 out]
                    n359 = Bundle By Name(cluster=w746, "Minimum"=0.0, "Maximum"=43200.0, "Increment"=3600.0) -> (w742:T14)
                    n360 = property on="Property Node" class="WFChart (strict)"(reference=w740, "XScale.Range"=w742) -> ()  [unwired: 1 in, 2 out]
                  }
                  frame True {
                    n361 = Multiply(x=w748, y=3600.0) -> (x*y=w747:dbl)
                    n362 = property on="Property Node" class="WFChart (strict)"(reference=w751) -> (reference out=w750:refnum<vi>, "XScale.Range"=w755:T14)  [unwired: 1 in, 1 out]
                    n363 = Bundle By Name(cluster=w755, "Minimum"=0.0, "Maximum"=w747, "Increment"=3600.0) -> (w752:T14)
                    n364 = property on="Property Node" class="WFChart (strict)"(reference=w750, "XScale.Range"=w752) -> ()  [unwired: 1 in, 2 out]
                  }
                }
              }
              frame 2 {
                n365 = Not Equal To 0?(x=w756) -> (x != 0?=w757:bool)
                n366 = case shown="True" w757 {
                  tunnel: w758 -> [w760 w768]
                  tunnel: w756 -> [_ w766]
                  frame False {
                    n367 = property on="Property Node" class="WFChart (strict)"(reference=w760) -> (reference out=w759:refnum<vi>, "XScale.Range"=w765:T14)  [unwired: 1 in, 1 out]
                    n368 = Bundle By Name(cluster=w765, "Minimum"=0.0, "Maximum"=60.0, "Increment"=1.0) -> (w761:T14)
                    n369 = property on="Property Node" class="WFChart (strict)"(reference=w759, "XScale.Range"=w761) -> ()  [unwired: 1 in, 2 out]
                  }
                  frame True {
                    n370 = property on="Property Node" class="WFChart (strict)"(reference=w768) -> (reference out=w767:refnum<vi>, "XScale.Range"=w772:T14)  [unwired: 1 in, 1 out]
                    n371 = Bundle By Name(cluster=w772, "Minimum"=0.0, "Maximum"=w766, "Increment"=1.0) -> (w769:T14)
                    n372 = property on="Property Node" class="WFChart (strict)"(reference=w767, "XScale.Range"=w769) -> ()  [unwired: 1 in, 2 out]
                  }
                }
              }
            }
          }
          event "Set Time TC Graph 4": Mouse Down {
            n373 = event-data() -> ()  [unwired: 1 in, 8 out]
            n374 = local read "Log/Linear Y-Axis 4"() -> (w774:u16)
            n375 = control-ref of="Custom Chart 4"() -> (w773:refnum<vi>)
            n376 = property on="Property Node" class="WFChart (strict)"(reference=w773, "YScale.Mapping Mode"=w774) -> ()  [unwired: 1 in, 2 out]
            n377 = local read "Total Time 4"() -> (w775:dbl)
            n378 = local read "Time Scale 4"() -> (w776:u16)
            n379 = case shown="2" w776 {
              tunnel: w773 -> [w781 w800 w819]
              tunnel: w775 -> [w779 w798 w817]
              frame 0, Default {
                n380 = Not Equal To 0?(x=w779) -> (x != 0?=w780:bool)
                n381 = case shown="True" w780 {
                  tunnel: w781 -> [w783 w795]
                  tunnel: w779 -> [_ w789]
                  frame False {
                    n382 = property on="Property Node" class="WFChart (strict)"(reference=w783) -> (reference out=w782:refnum<vi>, "XScale.Range"=w788:T14)  [unwired: 1 in, 1 out]
                    n383 = Bundle By Name(cluster=w788, "Minimum"=0.0, "Maximum"=3600.0, "Increment"=60.0) -> (w787:T14)
                    n384 = property on="Property Node" class="WFChart (strict)"(reference=w782, "XScale.Range"=w787) -> ()  [unwired: 1 in, 2 out]
                  }
                  frame True {
                    n385 = property on="Property Node" class="WFChart (strict)"(reference=w795) -> (reference out=w792:refnum<vi>, "XScale.Range"=w797:T14)  [unwired: 1 in, 1 out]
                    n386 = Multiply(x=w789, y=60.0) -> (x*y=w791:dbl)
                    n387 = Bundle By Name(cluster=w797, "Minimum"=0.0, "Maximum"=w791, "Increment"=1.0) -> (w796:T14)
                    n388 = property on="Property Node" class="WFChart (strict)"(reference=w792, "XScale.Range"=w796) -> ()  [unwired: 1 in, 2 out]
                  }
                }
              }
              frame 1 {
                n389 = Not Equal To 0?(x=w798) -> (x != 0?=w799:bool)
                n390 = case shown="True" w799 {
                  tunnel: w800 -> [w802 w812]
                  tunnel: w798 -> [_ w809]
                  frame False {
                    n391 = property on="Property Node" class="WFChart (strict)"(reference=w802) -> (reference out=w801:refnum<vi>, "XScale.Range"=w807:T14)  [unwired: 1 in, 1 out]
                    n392 = Bundle By Name(cluster=w807, "Minimum"=0.0, "Maximum"=43200.0, "Increment"=3600.0) -> (w803:T14)
                    n393 = property on="Property Node" class="WFChart (strict)"(reference=w801, "XScale.Range"=w803) -> ()  [unwired: 1 in, 2 out]
                  }
                  frame True {
                    n394 = Multiply(x=w809, y=3600.0) -> (x*y=w808:dbl)
                    n395 = property on="Property Node" class="WFChart (strict)"(reference=w812) -> (reference out=w811:refnum<vi>, "XScale.Range"=w816:T14)  [unwired: 1 in, 1 out]
                    n396 = Bundle By Name(cluster=w816, "Minimum"=0.0, "Maximum"=w808, "Increment"=3600.0) -> (w813:T14)
                    n397 = property on="Property Node" class="WFChart (strict)"(reference=w811, "XScale.Range"=w813) -> ()  [unwired: 1 in, 2 out]
                  }
                }
              }
              frame 2 {
                n398 = Not Equal To 0?(x=w817) -> (x != 0?=w818:bool)
                n399 = case shown="True" w818 {
                  tunnel: w819 -> [w821 w829]
                  tunnel: w817 -> [_ w827]
                  frame False {
                    n400 = property on="Property Node" class="WFChart (strict)"(reference=w821) -> (reference out=w820:refnum<vi>, "XScale.Range"=w826:T14)  [unwired: 1 in, 1 out]
                    n401 = Bundle By Name(cluster=w826, "Minimum"=0.0, "Maximum"=60.0, "Increment"=1.0) -> (w822:T14)
                    n402 = property on="Property Node" class="WFChart (strict)"(reference=w820, "XScale.Range"=w822) -> ()  [unwired: 1 in, 2 out]
                  }
                  frame True {
                    n403 = property on="Property Node" class="WFChart (strict)"(reference=w829) -> (reference out=w828:refnum<vi>, "XScale.Range"=w833:T14)  [unwired: 1 in, 1 out]
                    n404 = Bundle By Name(cluster=w833, "Minimum"=0.0, "Maximum"=w827, "Increment"=1.0) -> (w830:T14)
                    n405 = property on="Property Node" class="WFChart (strict)"(reference=w828, "XScale.Range"=w830) -> ()  [unwired: 1 in, 2 out]
                  }
                }
              }
            }
          }
          event "Set Time TC Graph 5": Mouse Down {
            n406 = event-data() -> ()  [unwired: 1 in, 8 out]
            n407 = local read "Log/Linear Y-Axis 5"() -> (w835:u16)
            n408 = control-ref of="Custom Chart 5"() -> (w834:refnum<vi>)
            n409 = property on="Property Node" class="WFChart (strict)"(reference=w834, "YScale.Mapping Mode"=w835) -> ()  [unwired: 1 in, 2 out]
            n410 = local read "Total Time 5"() -> (w836:dbl)
            n411 = local read "Time Scale 5"() -> (w837:u16)
            n412 = case shown="2" w837 {
              tunnel: w834 -> [w842 w861 w880]
              tunnel: w836 -> [w840 w859 w878]
              frame 0, Default {
                n413 = Not Equal To 0?(x=w840) -> (x != 0?=w841:bool)
                n414 = case shown="True" w841 {
                  tunnel: w842 -> [w844 w856]
                  tunnel: w840 -> [_ w850]
                  frame False {
                    n415 = property on="Property Node" class="WFChart (strict)"(reference=w844) -> (reference out=w843:refnum<vi>, "XScale.Range"=w849:T14)  [unwired: 1 in, 1 out]
                    n416 = Bundle By Name(cluster=w849, "Minimum"=0.0, "Maximum"=3600.0, "Increment"=60.0) -> (w848:T14)
                    n417 = property on="Property Node" class="WFChart (strict)"(reference=w843, "XScale.Range"=w848) -> ()  [unwired: 1 in, 2 out]
                  }
                  frame True {
                    n418 = property on="Property Node" class="WFChart (strict)"(reference=w856) -> (reference out=w853:refnum<vi>, "XScale.Range"=w858:T14)  [unwired: 1 in, 1 out]
                    n419 = Multiply(x=w850, y=60.0) -> (x*y=w852:dbl)
                    n420 = Bundle By Name(cluster=w858, "Minimum"=0.0, "Maximum"=w852, "Increment"=1.0) -> (w857:T14)
                    n421 = property on="Property Node" class="WFChart (strict)"(reference=w853, "XScale.Range"=w857) -> ()  [unwired: 1 in, 2 out]
                  }
                }
              }
              frame 1 {
                n422 = Not Equal To 0?(x=w859) -> (x != 0?=w860:bool)
                n423 = case shown="True" w860 {
                  tunnel: w861 -> [w863 w873]
                  tunnel: w859 -> [_ w870]
                  frame False {
                    n424 = property on="Property Node" class="WFChart (strict)"(reference=w863) -> (reference out=w862:refnum<vi>, "XScale.Range"=w868:T14)  [unwired: 1 in, 1 out]
                    n425 = Bundle By Name(cluster=w868, "Minimum"=0.0, "Maximum"=43200.0, "Increment"=3600.0) -> (w864:T14)
                    n426 = property on="Property Node" class="WFChart (strict)"(reference=w862, "XScale.Range"=w864) -> ()  [unwired: 1 in, 2 out]
                  }
                  frame True {
                    n427 = Multiply(x=w870, y=3600.0) -> (x*y=w869:dbl)
                    n428 = property on="Property Node" class="WFChart (strict)"(reference=w873) -> (reference out=w872:refnum<vi>, "XScale.Range"=w877:T14)  [unwired: 1 in, 1 out]
                    n429 = Bundle By Name(cluster=w877, "Minimum"=0.0, "Maximum"=w869, "Increment"=3600.0) -> (w874:T14)
                    n430 = property on="Property Node" class="WFChart (strict)"(reference=w872, "XScale.Range"=w874) -> ()  [unwired: 1 in, 2 out]
                  }
                }
              }
              frame 2 {
                n431 = Not Equal To 0?(x=w878) -> (x != 0?=w879:bool)
                n432 = case shown="True" w879 {
                  tunnel: w880 -> [w882 w890]
                  tunnel: w878 -> [_ w888]
                  frame False {
                    n433 = property on="Property Node" class="WFChart (strict)"(reference=w882) -> (reference out=w881:refnum<vi>, "XScale.Range"=w887:T14)  [unwired: 1 in, 1 out]
                    n434 = Bundle By Name(cluster=w887, "Minimum"=0.0, "Maximum"=60.0, "Increment"=1.0) -> (w883:T14)
                    n435 = property on="Property Node" class="WFChart (strict)"(reference=w881, "XScale.Range"=w883) -> ()  [unwired: 1 in, 2 out]
                  }
                  frame True {
                    n436 = property on="Property Node" class="WFChart (strict)"(reference=w890) -> (reference out=w889:refnum<vi>, "XScale.Range"=w894:T14)  [unwired: 1 in, 1 out]
                    n437 = Bundle By Name(cluster=w894, "Minimum"=0.0, "Maximum"=w888, "Increment"=1.0) -> (w891:T14)
                    n438 = property on="Property Node" class="WFChart (strict)"(reference=w889, "XScale.Range"=w891) -> ()  [unwired: 1 in, 2 out]
                  }
                }
              }
            }
          }
          event "Set Time TC Graph 6": Mouse Down {
            n439 = event-data() -> ()  [unwired: 1 in, 8 out]
            n440 = local read "Log/Linear Y-Axis 6"() -> (w896:u16)
            n441 = control-ref of="Custom Chart 6"() -> (w895:refnum<vi>)
            n442 = property on="Property Node" class="WFChart (strict)"(reference=w895, "YScale.Mapping Mode"=w896) -> ()  [unwired: 1 in, 2 out]
            n443 = local read "Total Time 6"() -> (w897:dbl)
            n444 = local read "Time Scale 6"() -> (w898:u16)
            n445 = case shown="2" w898 {
              tunnel: w895 -> [w903 w922 w941]
              tunnel: w897 -> [w901 w920 w939]
              frame 0, Default {
                n446 = Not Equal To 0?(x=w901) -> (x != 0?=w902:bool)
                n447 = case shown="True" w902 {
                  tunnel: w903 -> [w905 w917]
                  tunnel: w901 -> [_ w911]
                  frame False {
                    n448 = property on="Property Node" class="WFChart (strict)"(reference=w905) -> (reference out=w904:refnum<vi>, "XScale.Range"=w910:T14)  [unwired: 1 in, 1 out]
                    n449 = Bundle By Name(cluster=w910, "Minimum"=0.0, "Maximum"=3600.0, "Increment"=60.0) -> (w909:T14)
                    n450 = property on="Property Node" class="WFChart (strict)"(reference=w904, "XScale.Range"=w909) -> ()  [unwired: 1 in, 2 out]
                  }
                  frame True {
                    n451 = property on="Property Node" class="WFChart (strict)"(reference=w917) -> (reference out=w914:refnum<vi>, "XScale.Range"=w919:T14)  [unwired: 1 in, 1 out]
                    n452 = Multiply(x=w911, y=60.0) -> (x*y=w913:dbl)
                    n453 = Bundle By Name(cluster=w919, "Minimum"=0.0, "Maximum"=w913, "Increment"=1.0) -> (w918:T14)
                    n454 = property on="Property Node" class="WFChart (strict)"(reference=w914, "XScale.Range"=w918) -> ()  [unwired: 1 in, 2 out]
                  }
                }
              }
              frame 1 {
                n455 = Not Equal To 0?(x=w920) -> (x != 0?=w921:bool)
                n456 = case shown="True" w921 {
                  tunnel: w922 -> [w924 w934]
                  tunnel: w920 -> [_ w931]
                  frame False {
                    n457 = property on="Property Node" class="WFChart (strict)"(reference=w924) -> (reference out=w923:refnum<vi>, "XScale.Range"=w929:T14)  [unwired: 1 in, 1 out]
                    n458 = Bundle By Name(cluster=w929, "Minimum"=0.0, "Maximum"=43200.0, "Increment"=3600.0) -> (w925:T14)
                    n459 = property on="Property Node" class="WFChart (strict)"(reference=w923, "XScale.Range"=w925) -> ()  [unwired: 1 in, 2 out]
                  }
                  frame True {
                    n460 = Multiply(x=w931, y=3600.0) -> (x*y=w930:dbl)
                    n461 = property on="Property Node" class="WFChart (strict)"(reference=w934) -> (reference out=w933:refnum<vi>, "XScale.Range"=w938:T14)  [unwired: 1 in, 1 out]
                    n462 = Bundle By Name(cluster=w938, "Minimum"=0.0, "Maximum"=w930, "Increment"=3600.0) -> (w935:T14)
                    n463 = property on="Property Node" class="WFChart (strict)"(reference=w933, "XScale.Range"=w935) -> ()  [unwired: 1 in, 2 out]
                  }
                }
              }
              frame 2 {
                n464 = Not Equal To 0?(x=w939) -> (x != 0?=w940:bool)
                n465 = case shown="True" w940 {
                  tunnel: w941 -> [w943 w951]
                  tunnel: w939 -> [_ w949]
                  frame False {
                    n466 = property on="Property Node" class="WFChart (strict)"(reference=w943) -> (reference out=w942:refnum<vi>, "XScale.Range"=w948:T14)  [unwired: 1 in, 1 out]
                    n467 = Bundle By Name(cluster=w948, "Minimum"=0.0, "Maximum"=60.0, "Increment"=1.0) -> (w944:T14)
                    n468 = property on="Property Node" class="WFChart (strict)"(reference=w942, "XScale.Range"=w944) -> ()  [unwired: 1 in, 2 out]
                  }
                  frame True {
                    n469 = property on="Property Node" class="WFChart (strict)"(reference=w951) -> (reference out=w950:refnum<vi>, "XScale.Range"=w955:T14)  [unwired: 1 in, 1 out]
                    n470 = Bundle By Name(cluster=w955, "Minimum"=0.0, "Maximum"=w949, "Increment"=1.0) -> (w952:T14)
                    n471 = property on="Property Node" class="WFChart (strict)"(reference=w950, "XScale.Range"=w952) -> ()  [unwired: 1 in, 2 out]
                  }
                }
              }
            }
          }
          event "exit": Value Change {
            n472 = event-data() -> ()  [unwired: 1 in, 1 out]
            n473 = call "Broadcast Message.vi"("error in (no error)"=w958, "event"="exit") -> ("error out"=w956:errorcluster)  [unwired: 9 in]
          }
        }
      }
      frame "receivePressure" {
        n474 = Unflatten From JSON(JSON string=w960, type and defaults=T9 {"CryoPressure"=0.0, "ChamberPressure"=0.0, "RoughingPressure"=0.0}) -> (value=w966:T9)  [unwired: 5 in, 1 out]
        n475 = Unbundle By Name(w966) -> ("CryoPressure"=w965:dbl, "ChamberPressure"=w964:dbl, "RoughingPressure"=w963:dbl)
        n476 = Build Array(w965, w964, w963) -> (w967:dbl[])
        n477 = Bundle By Name(cluster=w969, "Pressure"=w967) -> (w968:T7)
      }
      frame "graphTC" {
        n478 = property on="Waveform Chart" class="WFChart (strict)"("LegScrollVis"=TRUE ("Legend:Scrollbar Visible")) -> ()  [unwired: 2 in, 2 out]
        n479 = Unbundle By Name(w980) -> ("working array"=w977:bool[], "Thermocouples"=w978:T3, "TCs"=w971:T4)
        n480 = for {
          N: 120 -> [_]
          tunnel: w971 -> [w1014] mode=indexing
          tunnel: [w1013] -> w972 mode=indexing
          shift-right: [w992] -> w974
          shift-left: w978 -> [w999]
          shift-right: [w991] -> w979
          shift-left: w977 -> [w990]
          i -> [w989]
          n481 = Unbundle By Name(w1014) -> ("thermocouple"=w1023:i32, "temp"=w987:dbl, "alarm"=w1018:i32, "working"=w1017:bool)
          n482 = Quotient & Remainder(x=w989, y=4) -> (x-y*floor(x/y)=w997:i32, floor(x/y)=w998:i32)
          n483 = Index Array(array=w999, index (row)=w998, index (col)=w997) -> (element=w1012:T8)
          n484 = Multiply(x=w998, y=4) -> (x*y=w1007:i32)
          n485 = Multiply(x=w998, y=4) -> (x*y=w1019:i32)
          n486 = Unbundle By Name(w1012) -> ("Graph On/Off"=w996:u32)
          n487 = Add(x=w1007, y=w997) -> (x+y=w1005:i32)
          n488 = Add(x=w1019, y=w997) -> (x+y=w988:i32)
          n489 = Replace Array Subset(array=w990, new element=w1017, index=w989) -> (w991:bool[])
          n490 = To Double Precision Float(number=w987) -> (double precision float=w986:dbl)
          n491 = Get Date/Time In Seconds() -> (seconds since 1Jan1904=w1016:timestamp)
          n492 = property on="Waveform Chart" class="WFChart (strict)"("Active Plot"=w988) -> ()  [unwired: 2 in, 2 out]
          n493 = Index Array(array=w991, index=w1005) -> (element=w1004:bool)
          n494 = Bundle By Name("t0"=w1016) -> (w1015:waveform(dbl))  [unwired: 1 in]
          n495 = Build Array(w986) -> (w985:dbl[])
          n496 = Number To Fractional String(number=w986, precision (6)=i16 2 ("width (-)")) -> (F-format string=w1002:string)  [unwired: 2 in]
          n497 = Bundle By Name(cluster=w1015, "Y"=w985) -> (w1013:waveform(dbl))
          n498 = case shown="True" w1004 {
            tunnel: w996 -> [_ w1028]
            tunnel: [u32 12369084 ("y") w1028] -> w1000
            tunnel: w1002 -> [_ w1027]
            tunnel: ["NaN" w1027] -> w1001
            frame False {
            }
            frame True {
            }
          }
          n499 = case shown="1" w1018 {
            tunnel: ["" "L" "H"] -> w993
            tunnel: w1018 -> [_ _ _]
            tunnel: [u32 12369084 u32 2812927 u32 16711680] -> w994
            frame 0, Default {
            }
            frame 1 {
            }
            frame 2 {
            }
          }
          n500 = Number To Decimal String(number=w1023) -> (decimal integer string=w1024:string)  [unwired: 1 in]
          n501 = Index Array(array=w999, index (row)=w998, index (col)=w997) -> (element=w1010:T8)
          n502 = Equal?(x=w1000, y=u32 6618880) -> (x = y?=w1008:bool)
          n503 = Concatenate Strings("TC " ("string"), w1024) -> (w995:string)
          n504 = property on="Waveform Chart" class="WFChart (strict)"("Plot.Plot Name"=w995) -> ()  [unwired: 2 in, 2 out]
          n505 = case shown="True" w1008 {
            tunnel: [w1036 w1044] -> w1011
            tunnel: w1010 -> [w1035 w1043]
            tunnel: w1000 -> [w1033 w1042]
            tunnel: w1001 -> [w1034 w1041]
            tunnel: w995 -> [w1032 w1040]
            tunnel: w994 -> [w1031 w1039]
            tunnel: w993 -> [w1030 w1038]
            frame False {
              n506 = Bundle By Name(cluster=w1035, "Graph On/Off"=w1033, "TC Label"=w1032, "PlotColor"=u32 12369084 ("y"), "Temperature"=w1034, "Alarm Color"=w1031, "Alarm Status"=w1030) -> (w1036:T8)
            }
            frame True {
              n507 = property on="Waveform Chart" class="WFChart (strict)"() -> ("Plot.Plot Color"=w1037:u32)  [unwired: 2 in, 2 out]
              n508 = Bundle By Name(cluster=w1043, "Graph On/Off"=w1042, "TC Label"=w1040, "PlotColor"=w1037, "Temperature"=w1041, "Alarm Color"=w1039, "Alarm Status"=w1038) -> (w1044:T8)
            }
          }
          n509 = Replace Array Subset(array=w999, new element=w1011, index (row)=w998, index (col)=w997) -> (w992:T3)
        }
        n510 = local write "Thermocouples"(w974) -> ()
        n511 = Bundle By Name(cluster=w980, "Thermocouples"=w974, "working array"=w979) -> (w975:T7)
        n512 = Build Array (concatenate)(waveform(dbl) {"t0"=timestamp(0 s since 1904-01-01), "dt"=1.0, "Y"=[]} ("element"), w972) -> (w983:waveform(dbl)[])
        n513 = Delete From Array(array=w983, index=0) -> (array with subset deleted=→"Waveform Chart":waveform(dbl)[])  [unwired: 1 in, 1 out]
      }
      frame "receiveTC" {
        n514 = Unflatten From JSON(JSON string=w1054, type and defaults=T10 {"time"="", "TCs"=[]} ("Cluster")) -> (value=w1057:T10)  [unwired: 5 in, 1 out]
        n515 = Unbundle By Name(w1057) -> ("TCs"=w1056:T4)
        n516 = Bundle By Name(cluster=w1055, "TCs"=w1056) -> (w1051:T7)
      }
      frame "receiveMCCData" {
        n517 = Unbundle By Name(w1073) -> ("Http session"=w1077:T6, "URL prefex"=w1075:string, "PumpTemps"=w1071:T5)
        n518 = Concatenate Strings(w1075, "getMCCData" ("url")) -> (w1076:string)
        n519 = call <vilib>:"GET.vi"("client handle"=w1077, "url"=w1076) -> ("body"=w1059:string)  [unwired: 10 in, 3 out]
        n520 = Unflatten From JSON(JSON string=w1059, type and defaults=T11 {"DutyCycle"=0, "Stage1Temp"=0, "CryoPumpReadyState"={"MotorOn"=FALSE, "Ready"=FALSE}, "PurgeValveState"=FALSE, "RegenError"="", "RegenStep"="", "RoughingValveState"=FALSE, "RoughingInterlock"={"RoughingPermission"=FALSE, "RoughingNeeded"=FALSE, "Cryopumprunning"=FALSE}, "Stage2Temp"=0, "Status"={"PumpOn"=FALSE, "RoughOpen"=FALSE, "PurgeOpen"=FALSE, "ThermocoupleGaugeOn"=FALSE, "PowerFailureOccurred"=FALSE}, "TcPressure"=0}) -> (value=w1070:T11)  [unwired: 5 in, 1 out]
        n521 = Unbundle By Name(w1070) -> ("Stage1Temp"=w1068:i32, "Stage2Temp"=w1067:i32, "TcPressure"=w1066:i32)
        n522 = To Double Precision Float(number=w1068) -> (double precision float=w1065:dbl)
        n523 = To Double Precision Float(number=w1067) -> (double precision float=w1064:dbl)
        n524 = To Double Precision Float(number=w1066) -> (double precision float=w1063:dbl)
        n525 = Build Array(w1064) -> (w1061:dbl[])
        n526 = Build Array(w1063) -> (w1062:dbl[])
        n527 = Build Array(w1065) -> (w1060:dbl[])
        n528 = Bundle(cluster=w1071, "Cp Stage 1 Temp"=w1060, "Cp Stage 2 Temp"=w1061, "Compressor Temp"=w1062) -> (w1072:T5)
        n529 = Bundle By Name(cluster=w1073, "PumpTemps"=w1072) -> (w1078:T7)
      }
      frame "getThermalProfile" {
        n530 = Unbundle By Name(w1082) -> ("Http session"=w1086:T6, "URL prefex"=w1084:string)
        n531 = local read "Local Debug"() -> (w1081:bool)
        n532 = case shown="True" "ThermalProfile" {
          tunnel: w1086 -> [_ w1096]
          tunnel: "getAllZoneData" ("url") -> [_ w1094]
          tunnel: w1084 -> [_ w1091]
          tunnel: cluster{"ZoneSetPoint":dbl[], "ZoneTemp":dbl[]} {"ZoneSetPoint"=[], "ZoneTemp"=[]} -> [_ w1090]
          tunnel: w1081 -> [_ w1089]
          frame False {
          }
          frame True {
            n533 = Flatten To JSON(anything=w1090) -> (JSON string=w1093:string)  [unwired: 2 in, 1 out]
            n534 = Concatenate Strings(w1091, w1094) -> (w1095:string)
            n535 = case shown="True" w1089 {
              tunnel: [w1101 w1102] -> _
              tunnel: [w1100 w1103] -> _
              tunnel: w1096 -> [_ _]
              tunnel: w1095 -> [w1099 w1106]
              tunnel: [w1098 w1104] -> w1092
              tunnel: [w1097 w1105] -> w1087
              tunnel: w1093 -> [_ w1107]
              frame False {
                n536 = call <vilib>:"GET.vi"("url"=w1099) -> ("client handle out"=w1100:T6, "headers"=w1097:string, "body"=w1098:string, "error out"=w1101:errorcluster)  [unwired: 11 in]
              }
              frame True {
                n537 = call-poly <vilib>:"POST.vi"("url"=w1106, "buffer"=w1107) -> ("client handle out"=w1103:T6, "headers"=w1105:string, "body"=w1104:string, "error out"=w1102:errorcluster)  [unwired: 10 in]
              }
            }
            "headers" <- w1087
            n538 = Unflatten From JSON(JSON string=w1092, type and defaults=w1090) -> (value=→"value":cluster{"ZoneSetPoint":dbl[], "ZoneTemp":dbl[]})  [unwired: 5 in, 1 out]
          }
        }
      }
      frame "getZones" {
        n539 = Unbundle By Name(w1118) -> ("Http session"=w1121:T6, "URL prefex"=w1116:string)
        n540 = Concatenate Strings(w1116, "getZoneTemps" ("url")) -> (w1120:string)
        n541 = local read "Local Debug"() -> (w1117:bool)
        n542 = case shown="True" "Read Zones" {
          tunnel: w1121 -> [_ w1132]
          tunnel: w1120 -> [_ w1131]
          tunnel: w1117 -> [_ w1128]
          tunnel: [_ w1125] -> w1112
          tunnel: [_ w1124] -> w1110
          frame False {
          }
          frame True {
            w1127 = cluster{"ZoneSetPoint":dbl[], "ZoneTemp":dbl[]} {"ZoneSetPoint"=[], "ZoneTemp"=[]}
            n543 = Flatten To JSON(anything=w1127) -> (JSON string=w1130:string)  [unwired: 2 in, 1 out]
            n544 = case shown="True" w1128 {
              tunnel: [w1137 w1138] -> _
              tunnel: [w1136 w1139] -> _
              tunnel: w1132 -> [_ _]
              tunnel: w1131 -> [w1135 w1142]
              tunnel: [w1134 w1140] -> w1129
              tunnel: [w1133 w1141] -> _
              tunnel: w1130 -> [_ w1143]
              frame False {
                n545 = call <vilib>:"GET.vi"("url"=w1135) -> ("client handle out"=w1136:T6, "headers"=w1133:string, "body"=w1134:string, "error out"=w1137:errorcluster)  [unwired: 11 in]
              }
              frame True {
                n546 = call-poly <vilib>:"POST.vi"("url"=w1142, "buffer"=w1143) -> ("client handle out"=w1139:T6, "headers"=w1141:string, "body"=w1140:string, "error out"=w1138:errorcluster)  [unwired: 10 in]
              }
            }
            n547 = Unflatten From JSON(JSON string=w1129, type and defaults=w1127) -> (value=w1126:cluster{"ZoneSetPoint":dbl[], "ZoneTemp":dbl[]})  [unwired: 5 in, 1 out]
            n548 = Unbundle By Name(w1126) -> ("ZoneSetPoint"=w1124:dbl[], "ZoneTemp"=w1125:dbl[])
          }
        }
        n549 = Initialize Array(0.0 ("element"), 18 ("dimension size")) -> (w1113:dbl[])
        n550 = for {
          N: 18 -> [_]
          tunnel: w1112 -> [w1145]
          shift-right: [w1144] -> w1109
          shift-left: w1113 -> [w1149]
          tunnel: w1110 -> [w1146]
          i -> [w1148]
          n551 = Quotient & Remainder(x=w1148, y=2) -> (x-y*floor(x/y)=w1147:i32)  [unwired: 1 out]
          n552 = Equal To 0?(x=w1147) -> (x = 0?=w1150:bool)
          n553 = case shown="False" w1150 {
            tunnel: w1149 -> [w1158 w1165]
            tunnel: w1148 -> [w1153 w1162]
            tunnel: [w1157 w1164] -> w1144
            tunnel: w1146 -> [w1154 _]
            tunnel: w1145 -> [_ w1163]
            frame False {
              n554 = Quotient & Remainder(x=w1153, y=2) -> (floor(x/y)=w1155:i32)  [unwired: 1 out]
              n555 = Index Array(array=w1154, index=w1155) -> (element=w1152:dbl)
              n556 = Replace Array Subset(array=w1158, new element=w1152, index=w1153) -> (w1157:dbl[])
            }
            frame True {
              n557 = Quotient & Remainder(x=w1162, y=2) -> (floor(x/y)=w1160:i32)  [unwired: 1 out]
              n558 = Index Array(array=w1163, index=w1160) -> (element=w1159:dbl)
              n559 = Replace Array Subset(array=w1165, new element=w1159, index=w1162) -> (w1164:dbl[])
            }
          }
        }
        n560 = Bundle By Name(cluster=w1118, "Zones"=w1109) -> (w1122:T7)
      }
      frame "masterDatabase" {
        n561 = Unbundle By Name(w1177) -> ("Thermocouples"=w1178:T3, "Pressure"=w1169:dbl[], "PumpTemps"=w1173:T5, "NumberTCs"=w1179:i32, "Zones"=w1166:dbl[])  [unwired: 1 out]
        n562 = Initialize Array(0.0 ("element"), w1179) -> (w1181:dbl[])
        n563 = Unbundle(w1173) -> ("Cp Stage 1 Temp"=w1172:dbl[], "Cp Stage 2 Temp"=w1171:dbl[], "Compressor Temp"=w1170:dbl[])
        n564 = Build Array (concatenate)(w1172, w1171, w1170) -> (w1168:dbl[])
        n565 = for {
          N: w1179 -> [_]
          shift-right: [w1191] -> w1167
          shift-left: w1181 -> [w1192]
          tunnel: w1178 -> [w1187]
          i -> [w1189]
          n566 = Quotient & Remainder(x=w1189, y=4) -> (x-y*floor(x/y)=w1186:i32, floor(x/y)=w1188:i32)
          n567 = Index Array(array=w1187, index (row)=w1188, index (col)=w1186) -> (element=w1185:T8)
          n568 = Unbundle By Name(w1185) -> ("Temperature"=w1184:string)
          n569 = Fract/Exp String To Number(string=w1184) -> (number=w1183:dbl)  [unwired: 3 in, 1 out]
          n570 = To Double Precision Float(number=w1183) -> (double precision float=w1193:dbl)
          n571 = Replace Array Subset(array=w1192, new element=w1193, index=w1189) -> (w1191:dbl[])
        }
        n572 = Build Array (concatenate)(dbl[] [0.0], w1169, w1166, w1167, w1168) -> (w1175:dbl[])
        n573 = Bundle By Name(cluster=w1177, "Database"=w1175) -> (w1176:T7)
      }
      frame "multipleGraphs" {
        n574 = local read "Custom Graph Selector"() -> (w1194:i32)
        n575 = for {
          N: 6 ("Numeric") -> [_]
          tunnel: w1197 -> [w1211]
          tunnel: w1196 -> [w1210]
          tunnel: w1194 -> [w1201]
          i -> [w1198]
          n576 = case shown="2" w1198 {
            tunnel: [w1257 w1258 w1260 w1262 w1264 w1266] -> w1203
            tunnel: [w1256 w1259 w1261 w1263 w1265 w1267] -> w1202
            frame 0, Default {
              n577 = control-ref of="Custom Chart 1 Selection"() -> (w1256:refnum<vi>)
              n578 = control-ref of="Custom Chart 1"() -> (w1257:refnum<vi>)
            }
            frame 1 {
              n579 = control-ref of="Custom Chart 2 Selection"() -> (w1259:refnum<vi>)
              n580 = control-ref of="Custom Chart 2"() -> (w1258:refnum<vi>)
            }
            frame 2 {
              n581 = control-ref of="Custom Chart 3 Selection"() -> (w1261:refnum<vi>)
              n582 = control-ref of="Custom Chart 3"() -> (w1260:refnum<vi>)
            }
            frame 3 {
              n583 = control-ref of="Custom Chart 4 Selection"() -> (w1263:refnum<vi>)
              n584 = control-ref of="Custom Chart 4"() -> (w1262:refnum<vi>)
            }
            frame 4 {
              n585 = control-ref of="Custom Chart 5 Selection"() -> (w1265:refnum<vi>)
              n586 = control-ref of="Custom Chart 5"() -> (w1264:refnum<vi>)
            }
            frame 5 {
              n587 = control-ref of="Custom Chart 6 Selection"() -> (w1267:refnum<vi>)
              n588 = control-ref of="Custom Chart 6"() -> (w1266:refnum<vi>)
            }
          }
          n589 = Equal?(x=w1201, y=w1198) -> (x = y?=w1199:bool)
          n590 = Unbundle By Name(w1210) -> ("Database"=w1208:dbl[], "numSensors"=w1209:i32)
          n591 = case shown="True" w1199 {
            tunnel: w1211 -> [_ w1225]
            tunnel: [w1214 w1219] -> w1207
            tunnel: [1000 w1218] -> w1206
            tunnel: w1202 -> [w1215 w1217]
            tunnel: [FALSE w1216] -> w1200
            frame False {
              n592 = property on="Property Node" class="LstBox (strict)"(reference=w1215) -> ("Item Symbols"=w1214:i32[])  [unwired: 1 in, 2 out]
            }
            frame True {
              n593 = property on="Property Node" class="LstBox (strict)"(reference=w1217) -> ("Item Symbols"=w1219:i32[])  [unwired: 1 in, 2 out]
              n594 = Decimal String To Number(string=w1225) -> (number=w1218:i32)  [unwired: 2 in, 1 out]
              n595 = Index Array(array=w1219, index=0) -> (element=w1220:i32)
              n596 = Equal?(x=37, y=w1220) -> (x = y?=w1222:bool)
              n597 = Equal To 0?(x=w1218) -> (x = 0?=w1224:bool)
              n598 = And(x=w1222, y=w1224) -> (x .and. y?=w1216:bool)
            }
          }
          n599 = case shown="True" w1200 {
            tunnel: [0 ("index") w1320] -> w1205
            tunnel: w1209 -> [w1274 w1316]
            tunnel: w1208 -> [w1273 _]
            tunnel: [w1272 _] -> w1204
            tunnel: w1206 -> [w1270 w1320]
            tunnel: w1207 -> [w1271 w1319]
            tunnel: w1202 -> [w1269 w1315]
            tunnel: w1203 -> [w1268 w1314]
            frame False {
              n600 = for {
                N: w1274 -> [_]
                tunnel: [w1293] -> w1272 mode=indexing
                tunnel: w1270 -> [w1287]
                tunnel: w1271 -> [w1282]
                tunnel: w1273 -> [w1279] mode=indexing
                tunnel: w1269 -> [w1277]
                tunnel: w1268 -> [w1276]
                i -> [w1280]
                n601 = Wait (ms)(milliseconds to wait=u32 0) -> ()  [unwired: 1 out]
                n602 = Get Date/Time In Seconds() -> (seconds since 1Jan1904=w1295:timestamp)
                n603 = Bundle By Name("t0"=w1295) -> (w1294:waveform(dbl))  [unwired: 1 in]
                n604 = Build Array(w1279) -> (w1278:dbl[])
                n605 = Bundle By Name(cluster=w1294, "Y"=w1278) -> (w1293:waveform(dbl))
                n606 = Index Array(array=w1282, index=w1287) -> (element=w1285:i32)
                n607 = Index Array(array=w1282, index=w1287) -> (element=w1288:i32)
                n608 = Equal?(x=w1285, y=38) -> (x = y?=w1284:bool)
                n609 = Equal?(x=w1288, y=37) -> (x = y?=w1290:bool)
                n610 = Equal?(x=w1280, y=w1287) -> (x = y?=w1283:bool)
                n611 = And(x=w1283, y=w1284) -> (x .and. y?=w1281:bool)
                n612 = And(x=w1283, y=w1290) -> (x .and. y?=w1289:bool)
                n613 = case shown="True" w1289 {
                  tunnel: w1282 -> [_ w1313]
                  tunnel: w1287 -> [_ _]
                  tunnel: w1280 -> [_ w1308]
                  tunnel: w1276 -> [_ w1305]
                  tunnel: w1277 -> [_ w1306]
                  frame False {
                  }
                  frame True {
                    n614 = property on="Property Node" class="WFChart (strict)"(reference=w1305, "Active Plot"=w1308) -> (reference out=w1311:refnum<vi>)  [unwired: 1 in, 1 out]
                    n615 = Replace Array Subset(array=w1313, new element=38, index=w1308) -> (w1309:i32[])
                    n616 = property on="Property Node" class="WFChart (strict)"(reference=w1305) -> ("Plot.Plot Color"=w1307:u32)  [unwired: 1 in, 2 out]
                    n617 = property on="Property Node" class="WFChart (strict)"(reference=w1311, "Plot.Visible?"=TRUE ("Plot.Visible")) -> ()  [unwired: 1 in, 2 out]
                    n618 = property on="Property Node" class="LstBox (strict)"(reference=w1306, "Active Row"=w1308) -> ()  [unwired: 1 in, 2 out]
                    n619 = property on="Property Node" class="LstBox (strict)"(reference=w1306, "CellBG"=w1307) -> ()  [unwired: 1 in, 2 out]
                    n620 = property on="Property Node" class="LstBox (strict)"(reference=w1306, "Item Symbols"=w1309) -> ()  [unwired: 1 in, 2 out]
                  }
                }
                n621 = case shown="True" w1281 {
                  tunnel: w1282 -> [_ w1304]
                  tunnel: w1280 -> [_ w1297]
                  tunnel: w1276 -> [_ w1298]
                  tunnel: w1277 -> [_ w1299]
                  frame False {
                  }
                  frame True {
                    n622 = property on="Property Node" class="WFChart (strict)"(reference=w1298, "Active Plot"=w1297) -> (reference out=w1302:refnum<vi>)  [unwired: 1 in, 1 out]
                    n623 = Replace Array Subset(array=w1304, new element=37, index=w1297) -> (w1300:i32[])
                    n624 = property on="Property Node" class="WFChart (strict)"(reference=w1302, "Plot.Visible?"=FALSE ("Plot.Visible")) -> ()  [unwired: 1 in, 2 out]
                    n625 = property on="Property Node" class="LstBox (strict)"(reference=w1299, "Active Row"=w1297) -> ()  [unwired: 1 in, 2 out]
                    n626 = property on="Property Node" class="LstBox (strict)"(reference=w1299, "CellBG"=u32 13816530 ("Active Row:Cell Background Color")) -> ()  [unwired: 1 in, 2 out]
                    n627 = property on="Property Node" class="LstBox (strict)"(reference=w1299, "Item Symbols"=w1300) -> ()  [unwired: 1 in, 2 out]
                  }
                }
              }
            }
            frame True {
              n628 = for {
                N: w1316 -> [_]
                tunnel: w1319 -> [_]
                tunnel: w1315 -> [w1322]
                tunnel: w1314 -> [w1321]
                i -> [w1323]
                n629 = property on="Property Node" class="WFChart (strict)"(reference=w1321, "Active Plot"=w1323) -> (reference out=w1326:refnum<vi>)  [unwired: 1 in, 1 out]
                n630 = property on="Property Node" class="WFChart (strict)"(reference=w1326, "Plot.Visible?"=FALSE ("Plot.Visible")) -> ()  [unwired: 1 in, 2 out]
                n631 = property on="Property Node" class="LstBox (strict)"(reference=w1322, "Active Row"=w1323) -> ()  [unwired: 1 in, 2 out]
                n632 = property on="Property Node" class="LstBox (strict)"(reference=w1322, "CellBG"=u32 13816530 ("Active Row:Cell Background Color")) -> ()  [unwired: 1 in, 2 out]
              }
              n633 = Initialize Array(37, w1316) -> (w1317:i32[])
              n634 = property on="Property Node" class="LstBox (strict)"(reference=w1315, "Item Symbols"=w1317) -> ()  [unwired: 1 in, 2 out]
            }
          }
          n635 = case shown="5" w1198 {
            tunnel: w1205 -> [w1227 w1232 w1237 w1242 w1247 w1252]
            tunnel: w1204 -> [w1226 w1231 w1236 w1241 w1246 w1251]
            frame 0, Default {
              n636 = Build Array (concatenate)(waveform(dbl) {"t0"=timestamp(0 s since 1904-01-01), "dt"=1.0, "Y"=[]} ("element"), w1226) -> (w1230:waveform(dbl)[])
              n637 = Delete From Array(array=w1230, index=w1227) -> (array with subset deleted=→"Custom Chart 1":waveform(dbl)[])  [unwired: 1 in, 1 out]
            }
            frame 1 {
              n638 = Build Array (concatenate)(waveform(dbl) {"t0"=timestamp(0 s since 1904-01-01), "dt"=1.0, "Y"=[]} ("element"), w1231) -> (w1235:waveform(dbl)[])
              n639 = Delete From Array(array=w1235, index=w1232) -> (array with subset deleted=→"Custom Chart 2":waveform(dbl)[])  [unwired: 1 in, 1 out]
            }
            frame 2 {
              n640 = Build Array (concatenate)(waveform(dbl) {"t0"=timestamp(0 s since 1904-01-01), "dt"=1.0, "Y"=[]} ("element"), w1236) -> (w1240:waveform(dbl)[])
              n641 = Delete From Array(array=w1240, index=w1237) -> (array with subset deleted=→"Custom Chart 3":waveform(dbl)[])  [unwired: 1 in, 1 out]
            }
            frame 3 {
              n642 = Build Array (concatenate)(waveform(dbl) {"t0"=timestamp(0 s since 1904-01-01), "dt"=1.0, "Y"=[]} ("element"), w1241) -> (w1245:waveform(dbl)[])
              n643 = Delete From Array(array=w1245, index=w1242) -> (array with subset deleted=→"Custom Chart 4":waveform(dbl)[])  [unwired: 1 in, 1 out]
            }
            frame 4 {
              n644 = Build Array (concatenate)(waveform(dbl) {"t0"=timestamp(0 s since 1904-01-01), "dt"=1.0, "Y"=[]} ("element"), w1246) -> (w1250:waveform(dbl)[])
              n645 = Delete From Array(array=w1250, index=w1247) -> (array with subset deleted=→"Custom Chart 5":waveform(dbl)[])  [unwired: 1 in, 1 out]
            }
            frame 5 {
              n646 = Build Array (concatenate)(waveform(dbl) {"t0"=timestamp(0 s since 1904-01-01), "dt"=1.0, "Y"=[]} ("element"), w1251) -> (w1255:waveform(dbl)[])
              n647 = Delete From Array(array=w1255, index=w1252) -> (array with subset deleted=→"Custom Chart 6":waveform(dbl)[])  [unwired: 1 in, 1 out]
            }
          }
        }
      }
      frame "setThermalProfile" {
        n648 = event shown="[0] \"Set Z 1\": Mouse Down" {
          selector: _ -> [_]
          dyn-events: _ -> [_]
          timeout: _ -> [_]
          tunnel: T2 {"profiles"=[]} -> [w1336]
          event "Set Z 1": Mouse Down {
            n649 = event-data() -> ()  [unwired: 1 in, 8 out]
            n650 = local read "Cluster"() -> (w1330:T2)
            n651 = Unbundle By Name(w1330) -> ("profiles"=w1331:T15)
            n652 = Array To Cluster(array=w1331) -> (cluster=w1335:T16)
            n653 = local read "Zone 1 Temp"() -> (w1333:u16)
            n654 = Unbundle By Name(w1335) -> ("profiles[0]"=w1334:T1)
            n655 = Bundle By Name(cluster=w1334, "zone"=1, "average"=w1333) -> (→"output cluster":T1)
            "Cluster" <- w1336
          }
        }
      }
      frame "exit" {
        n656 = Unbundle By Name(w1338) -> ("Http session"=w1339:T6)
        n657 = call <vilib>:"CloseHandle.vi"("client handle"=w1339, "error in (no error)"=w1341) -> ("error out"=w1340:errorcluster)  [unwired: 13 in]
        n658 = Bundle By Name(cluster=w1338, "go"=FALSE ("Bundle Element")) -> (w1342:T7)
      }
      frame Default {
        n659 = call "Unknown Message Dialog.vi"("error in (no error)"=w1345, "event name"=w1344) -> ("error out"=w1343:errorcluster)  [unwired: 9 in]
      }
    }
    n660 = Unbundle By Name(w32) -> ("go"=w31:bool)
    n661 = call "log system event.vi"("error in (no error)"=w34) -> ("error out"=w33:errorcluster)  [unwired: 9 in, 1 out]
  }
  n662 = call "Unload Module.vi"("error in (no error)"=w11) -> ()  [unwired: 10 in, 1 out]
  n663 = property on="Waveform Chart" class="WFChart (strict)" props=["Plot", "Visible?"]() -> ()  [unwired: 2 in, 3 out]
